vi "DHE_Settings.vi"(0 "refnum":i32, 1 "DHE_DBSRef":T1, 2 "raw args":string, 5 "Command":string, 7 "physical unit":string, 11 "error in (no error)":errorcluster, 12 "switches":string[](array[string]), 13 "switches args":string[](array[string])) -> (3 "message":string, 4 "refnum out":i32, 8 "Read Value":i32, 15 "error out":errorcluster)   [LabVIEW 2016]
uses:
  DBSHAND/private/vis/DatabaseHand_RefNum.ctl
  DBSHAND/private/vis/DatabaseHand_Element_Set(string).vi
  DBSHAND/private/vis/DatabaseHand_Element_Set(U32).vi
  DBSHAND/private/vis/DatabaseHand_Element_Set(bool).vi
  DBSHAND/private/vis/DatabaseHand_Element_Get(U16).vi
  DBSHAND/private/vis/DatabaseHand_Element_Set(U16).vi
  DBSHAND/private/vis/DatabaseHand_Element_Get(bool).vi
  DBSHAND/private/vis/DatabaseHand_Element_Set(double).vi
  DBSHAND/private/vis/DatabaseHand_Element_Set(I32).vi
  DBSHAND/private/vis/DatabaseHand_Element_Get(string).vi
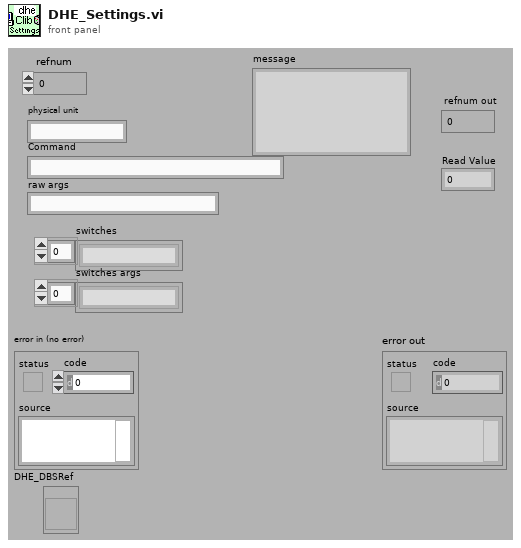
[diagram p1: front panel]
types:
  T1 = typedef "DatabaseHand_RefNum.ctl" = refnum<vi>
  T2 = enum16{"get", "send", "delete", "add", "clean", "send_all", "send_on", "send_off"}
  T3 = enum16{"add", "delete", "find", "clear all", "getall", "all"}
  T4 = enum16{"add", "delete", "find", "clear all", "getall"}
  T5 = typedef "CMN_ContStatus.ctl" = cluster{"Response":string, "power":bool, "shutter":bool, "artifdata":bool, "idlemode":bool, "reset":bool, "gain":u8, "speed":u8, "resetPCI":bool, "autoshutter":bool, "TempSetPoint":i32, "multipleextensions":bool, "displayImage":bool, "coadding":bool, "images being coadded":i32, "Operation Mode":enum16{"normal", "coadd", "fawler"}, "frames to write":cluster{"subs":bool, "reset":bool, "exposed":bool}, "fawler samples":i32, "write auto":bool, "datatype":string, "frames to display":cluster{"subs":bool, "reset":bool, "exposed":bool}, "sur":i32, "autoclear":bool}
  T6 = typedef "DHE_Img.ctl" = cluster{"title":string, "comment":string, "rootname":string, "imnumber":i32, "mext":bool, "imdir":string, "basename":string, "imprefix":string, "imsufix":string, "froot":string}
  T7 = typedef "DHE_Obs.ctl" = cluster{"observer":string, "obstype":string, "exptime":dbl, "coadds":i32, "fowler":i32, "nimages":i32, "display":bool, "autowrite":bool, "frames to write":cluster{"subs":bool, "reset":bool, "exposed":bool}, "frames to display":cluster{"subs":bool, "reset":bool, "exposed":bool}, "sur":i32}
  T8 = typedef "CMN_TimingInfo.ctl" = cluster{"PixelTime":sgl, "SkipPixel":sgl, "SkipRow":sgl, "ShiftRow":sgl, "ShiftedPix":u16, "known_overhead":sgl, "DET_READ_TIME":sgl}
  T9 = typedef "GEOM_CorrectedFPA.ctl" = cluster{"readmode":string, "amplifiers":cluster{"number":i32, "xstart":i32, "ystart":i32}[], "totxsize":i32, "totysize":i32, "maxxdim":i32, "maxydim":i32, "numxamps":i32, "numyamps":i32, "totxdata":i32, "totydata":i32, "xdataamp":i32, "ydataamp":i32, "totpixels":i32}
  T10 = typedef "GEOM_Amplifier.ctl" = cluster{"number":i32, "type":T11, "rotated":i16, "fliped":u16, "FPAcoord":cluster{"xstart":i32, "ystart":i32}, "Physical_size":cluster{"columns":i32, "rows":i32}, "predata":cluster{"columns":i32, "rows":i32}, "postdata":cluster{"columns":i32, "rows":i32}, "Req ROIs":T12, "Corr ROI":T12, "Detnumber":i32, "ampID":string, "discard":i32}
  T11 = typedef "GEOM_AmpType.ctl" = u16
  T12 = typedef "GEOM_ROI.ctl" = T13[]
  T13 = typedef "GEOM_Coords.ctl" = cluster{"xstart":u32, "ystart":u32, "xsize":u32, "ysize":u32}
  T14 = typedef "GEOM_AmpModifiers.ctl" = cluster{"Binning":T15, "sections":T16[]}
  T15 = typedef "GEOM_Binning.ctl" = cluster{"x":u32, "y":u32}
  T16 = typedef "GEOM_Moifier.ctl" = cluster{"name":string, "header section":string, "comment":string, "value":i32, "binning?":bool, "Where":enum16{"predata", "postdata"}, "add In":enum16{"columns", "rows", "none"}}
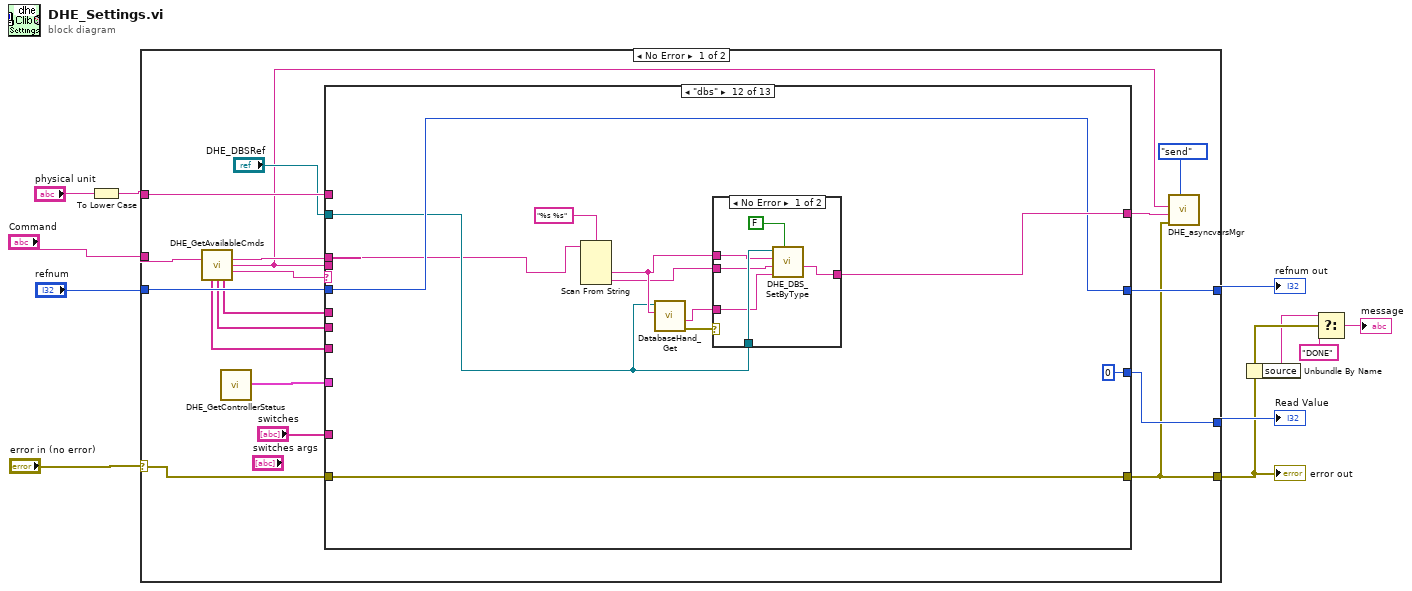
[diagram p0: block diagram]
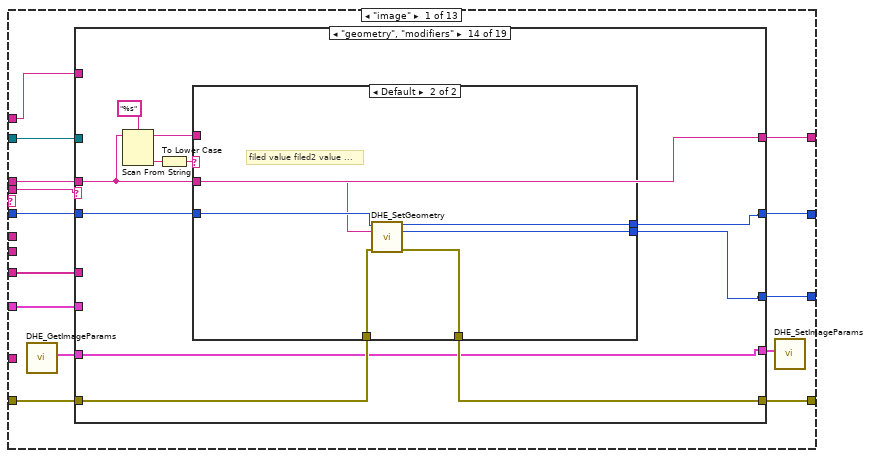
[diagram p2: hidden frame]
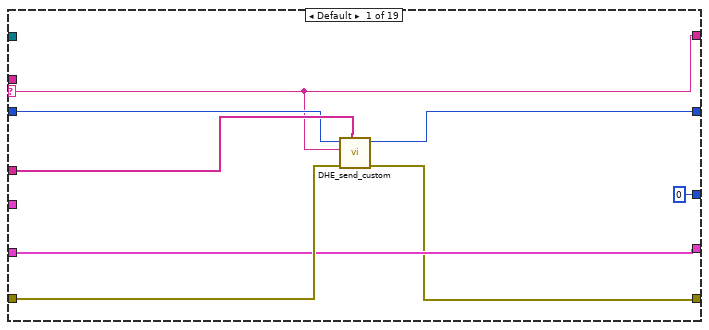
[diagram p3: hidden frame]
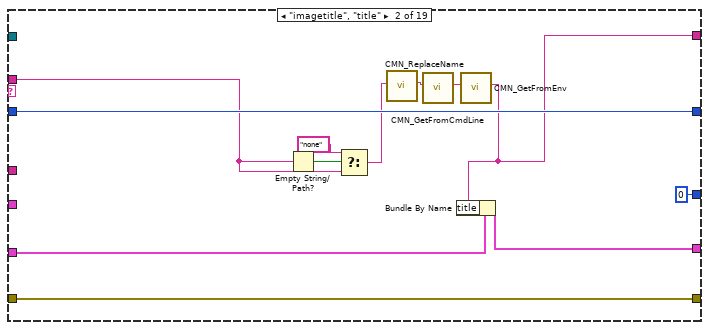
[diagram p4: hidden frame]
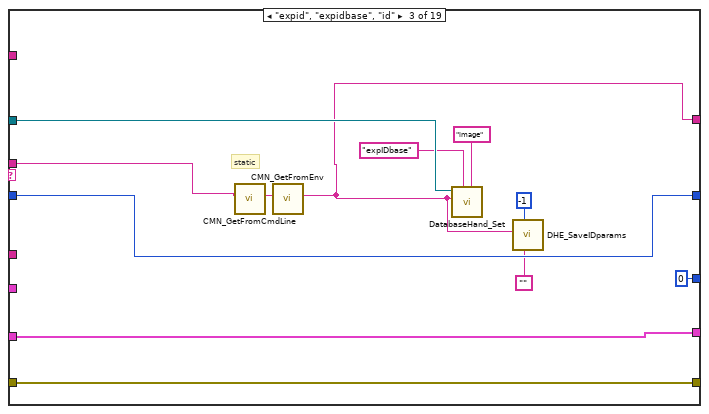
[diagram p5: hidden frame]
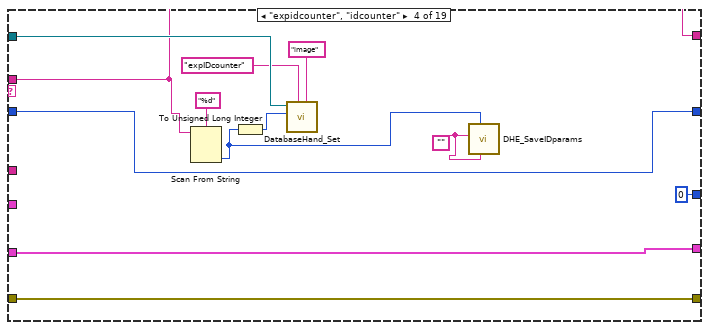
[diagram p6: hidden frame]
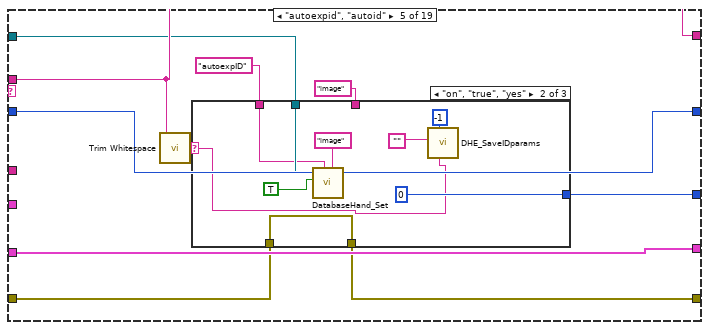
[diagram p7: hidden frame]
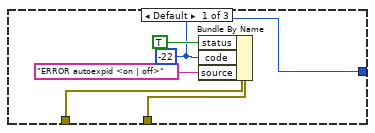
[diagram p8: hidden frame]
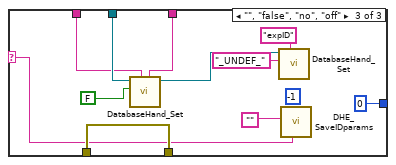
[diagram p9: hidden frame]
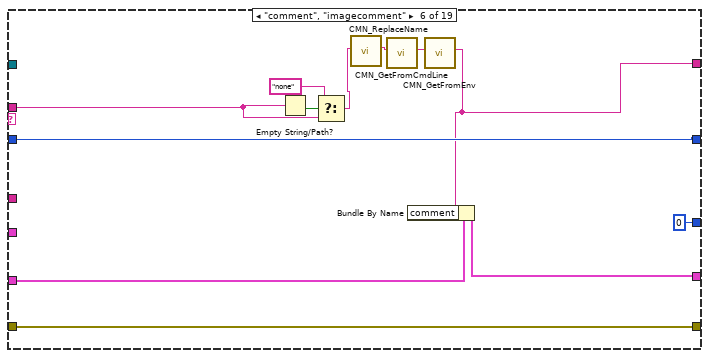
[diagram p10: hidden frame]
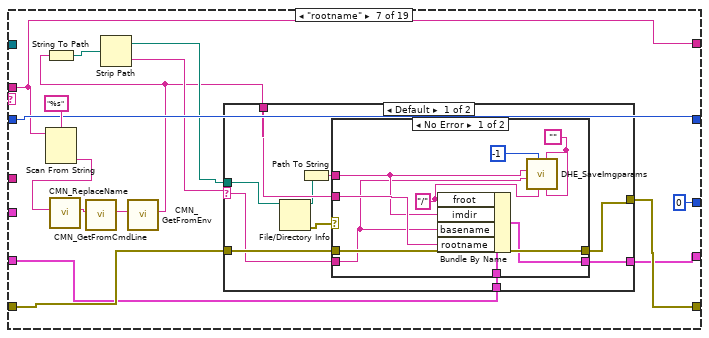
[diagram p11: hidden frame]
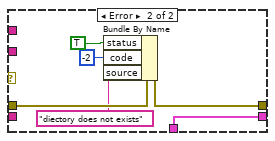
[diagram p12: hidden frame]
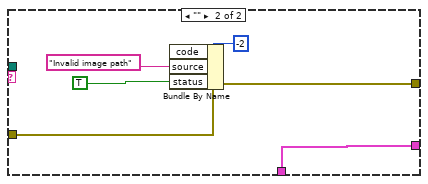
[diagram p13: hidden frame]
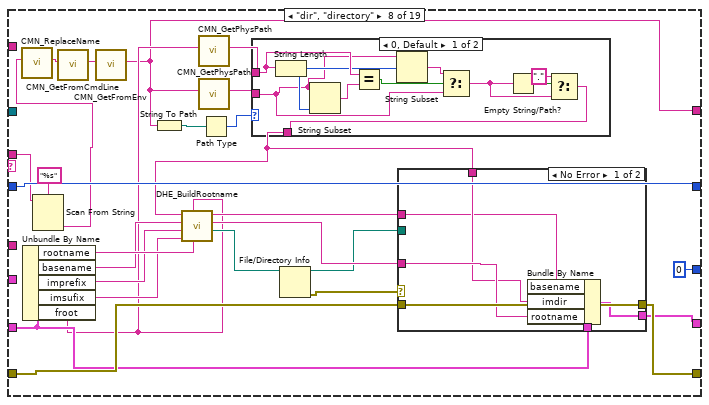
[diagram p14: hidden frame]
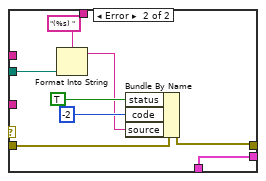
[diagram p16: hidden frame]
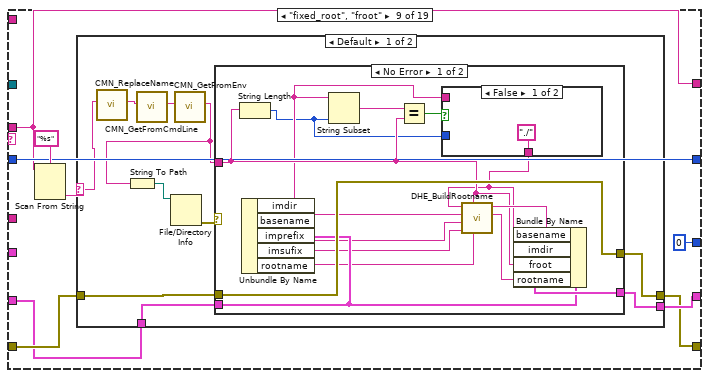
[diagram p17: hidden frame]
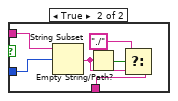
[diagram p18: hidden frame]
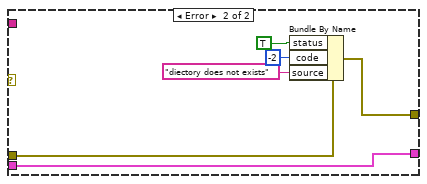
[diagram p19: hidden frame]
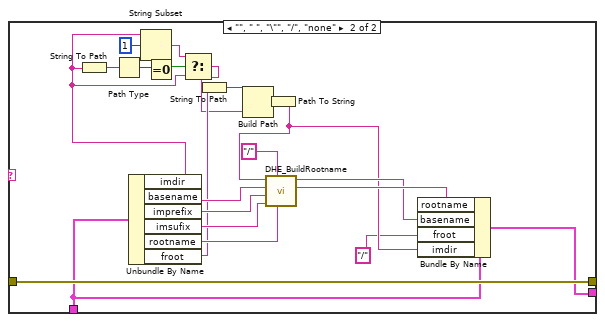
[diagram p20: hidden frame]
diagram:
  n1 = To Lower Case(string="physical unit") -> (all lower case string=w6:string)
  n2 = case shown="No Error" "error in (no error)" {
    selector: "error in (no error)" -> [w24 w2013]
    tunnel: [w14 w2013] -> w4
    tunnel: "refnum" -> [w29 w2015]
    tunnel: [w28 w2015] -> w10
    tunnel: "Command" -> [w23 _]
    tunnel: [w27 w2014] -> w11
    tunnel: w6 -> [w25 _]
    frame No Error {
      n3 = call "DHE_GetAvailableCmds.vi"("input command"=w23) -> ("remaining"=w18:string, "field"=w13:string, "parent"=w19:string, "SDSU_image_cmds out"=w20:string[], "SDSU_dhe_cmds out"=w21:string[], "SDSU_obs_cmds out"=w22:string[])  [unwired: 9 out]
      n4 = call "DHE_GetControllerStatus.vi"() -> ("ControllerStatus"=w26:T5)  [unwired: 11 out]
      n5 = case shown="\"dbs\"" w19 {
        selector: w19 -> [_ _ _ _ _ _ _ _ _ _ _ _ w1992]
        tunnel: w24 -> [w40 w617 w1252 w1806 w1831 w1833 w1843 w1854 w1889 w1940 w1942 w1974 w1999]
        tunnel: [w39 w609 w1248 w1805 w1831 w1833 w1843 w1853 w1885 w1940 w1941 w1974 w1989] -> w14
        tunnel: w29 -> [w38 w619 w1251 w1803 w1830 w1834 w1844 w1851 w1891 w1939 w1950 w1975 w1996]
        tunnel: [w37 w618 w1250 w1803 w1830 w1834 w1844 w1851 w1887 w1939 w1950 w1975 w1995] -> w28
        tunnel: [w43 w620 w1249 w1804 u32 0 ("code") u32 0 ("code") u32 0 ("code") w1852 w1886 u32 0 ("code") u32 0 ("code") u32 0 ("code") w1998] -> w27
        tunnel: w18 -> [w42 w621 w1247 w1808 w1827 w1836 w1846 w1850 w1883 w1935 w1948 w1971 w1994]
        tunnel: w26 -> [w35 w614 w1244 w1800 _ _ _ _ _ _ _ _ _]
        tunnel: w25 -> [w30 w615 _ _ _ _ _ _ _ _ _ _ _]
        tunnel: w22 -> [_ w616 _ _ _ _ _ _ _ _ _ _ _]
        tunnel: w21 -> [_ _ w1245 _ _ _ _ _ _ _ _ _ _]
        tunnel: w20 -> [w36 _ _ _ _ _ _ _ _ _ _ _ _]
        tunnel: w13 -> [w41 w610 w1246 _ _ _ _ _ _ _ _ _ _]
        tunnel: "DHE_DBSRef" -> [w31 w611 w1243 _ _ _ _ w1855 w1890 w1932 _ w1972 _]
        tunnel: "switches" -> [_ w607 _ _ _ _ _ _ w1884 _ _ _ _]
        tunnel: [w32 w608 w1242 w1799 "" w1832 w1842 w1850 w1883 w1935 w1943 w1976 w1992] -> w12
        frame "image" {
          n6 = call "DHE_GetImageParams.vi"() -> ("DHE_IMAGE"=w34:T6)  [unwired: 11 out]
          n7 = case shown="\"geometry\", \"modifiers\"" w41 {
            selector: w41 -> [w44 _ _ _ _ _ _ _ _ _ _ _ _ _ _ _ _ _ _]
            tunnel: [u32 0 ("code") u32 0 ("code") u32 0 ("code") u32 0 ("code") w89 u32 0 ("code") u32 0 ("code") u32 0 ("code") u32 0 ("code") u32 0 ("code") u32 0 ("code") u32 0 ("code") u32 0 ("code") w412 w437 w452 w493 w530 u32 0 ("code")] -> w43
            tunnel: w42 -> [_ w56 w64 w80 w95 w125 w139 w185 w233 w306 w348 w379 w400 w410 _ w449 w491 w534 w594]
            tunnel: w40 -> [w51 w62 w74 w86 w92 w134 w146 w205 w239 w320 w351 w382 w405 w416 w439 w444 w486 w532 w592]
            tunnel: [w45 w62 w74 w86 w91 w134 w145 w204 w234 w319 w350 w381 w405 w415 w438 w443 w485 w531 w592] -> w39
            tunnel: w38 -> [w47 w61 w72 w84 w97 w132 w147 w206 w237 w321 w352 w383 w403 w414 w436 w451 w492 w528 w589]
            tunnel: [w46 w61 w72 w84 w97 w132 w147 w206 w237 w321 w352 w383 w403 w413 w436 w451 w492 w529 w589] -> w37
            tunnel: w36 -> [w49 _ _ _ _ _ _ _ _ _ _ _ _ _ _ _ _ _ _]
            tunnel: w35 -> [_ _ _ _ _ _ _ _ _ _ _ _ _ _ _ w453 _ _ _]
            tunnel: w34 -> [w48 w60 w69 w81 w96 w131 w143 w201 w238 w316 w346 w377 w402 w411 w435 w448 w488 w527 w591]
            tunnel: [w48 w59 w69 w81 w96 w130 w142 w202 w235 w317 w347 w378 w401 w411 w435 w450 w488 w527 w591] -> w33
            tunnel: [w44 w52 w67 w80 w95 w123 w139 w181 w233 w302 w334 w365 w400 w410 "" ("remaining") w442 w490 w533 w588] -> w32
            tunnel: w31 -> [_ _ w71 w83 w94 _ _ _ _ _ _ _ _ _ _ w445 w489 w536 w585]
            tunnel: w30 -> [_ _ _ _ _ _ _ _ _ _ _ _ _ _ _ _ _ w535 w593]
            frame Default {
              n8 = call "DHE_send_custom.vi"("valid params"=w49, "error in (no error)"=w51, "args"=w44, "fd"=w47) -> ("error IO"=w45:errorcluster, "fd out"=w46:i32)  [unwired: 6 out]
            }
            frame "imagetitle", "title" {
              n9 = Empty String/Path?(string/path=w56) -> (empty?=w58:bool)
              n10 = Select(t="none", s=w58, f=w56) -> (s? t:f=w53:string)
              n11 = call "CMN_ReplaceName.vi"("name in"=w53) -> ("name out"=w54:string)  [unwired: 1 in, 9 out]
              n12 = call "CMN_GetFromCmdLine.vi"("str in"=w54) -> ("str out"=w55:string)  [unwired: 10 out]
              n13 = call "CMN_GetFromEnv.vi"("str in"=w55) -> ("str out"=w52:string)  [unwired: 10 out]
              n14 = Bundle By Name(cluster=w60, "title"=w52) -> (w59:T6)
            }
            frame "expid", "expidbase", "id" {
              # "static"
              n15 = call "CMN_GetFromCmdLine.vi"("str in"=w64) -> ("str out"=w68:string)  [unwired: 10 out]
              n16 = call "CMN_GetFromEnv.vi"("str in"=w68) -> ("str out"=w67:string)  [unwired: 10 out]
              n17 = call-poly "DatabaseHand_Set.vi"("group"="image", "name"="expIDbase" ("value"), "value"=w67, "Database RefNum in"=w71) -> ()  [unwired: 4 in, 4 out]
              n18 = call "DHE_SaveIDparams.vi"("autoid"="", "expidcounter"=-1, "expidbase"=w67) -> ()  [unwired: 9 out]
            }
            frame "expidcounter", "idcounter" {
              w78 = ""
              n19 = Scan From String(format string="%d", input string=w80) -> (output 1=w76:i32)  [unwired: 2 in, 4 out]
              n20 = To Unsigned Long Integer(number=w76) -> (unsigned 32bit integer=w77:u32)
              n21 = call-poly "DatabaseHand_Set.vi"("group"="image", "name"="expIDcounter" ("value"), "value"=w77, "Database RefNum in"=w83) -> ()  [unwired: 4 in, 4 out]
              n22 = call "DHE_SaveIDparams.vi"("autoid"=w78, "expidcounter"=w76, "expidbase"=w78) -> ()  [unwired: 9 out]
            }
            frame "autoexpid", "autoid" {
              n23 = call <vilib>:"Trim Whitespace.vi"("string"=w95) -> ("trimmed string"=w88:string)  [unwired: 1 in]
              n24 = case shown="\"on\", \"true\", \"yes\"" w88 {
                selector: w88 -> [_ w104 w112]
                tunnel: w94 -> [_ w110 w122]
                tunnel: "autoexpID" ("value") -> [_ w108 w120]
                tunnel: w92 -> [w102 w107 w119]
                tunnel: [w101 w107 w119] -> w91
                tunnel: "image" ("group") -> [_ _ w118]
                tunnel: [w98 0 ("code") 0 ("code")] -> w89
                frame Default {
                  w98 = -22 ("code")
                  n25 = Bundle By Name(cluster=w102, "status"=TRUE, "code"=w98, "source"="ERROR autoexpid <on | off>") -> (w101:errorcluster)
                }
                frame "on", "true", "yes" {
                  n26 = call-poly "DatabaseHand_Set.vi"("group"="image", "name"=w108, "value"=TRUE, "Database RefNum in"=w110) -> ()  [unwired: 4 in, 4 out]
                  n27 = call "DHE_SaveIDparams.vi"("autoid"=w104, "expidcounter"=-1, "expidbase"="") -> ()  [unwired: 9 out]
                }
                frame "", "false", "no", "off" {
                  (unwired) -1 ("expidcounter")
                  n28 = call-poly "DatabaseHand_Set.vi"("group"=w118, "name"=w120, "value"=FALSE, "Database RefNum in"=w122) -> ("Database RefNum out"=w116:T1)  [unwired: 4 in, 3 out]
                  n29 = call-poly "DatabaseHand_Set.vi"("name"="expID", "value"="_UNDEF_", "Database RefNum in"=w116) -> ()  [unwired: 5 in, 4 out]
                  n30 = call "DHE_SaveIDparams.vi"("autoid"=w112, "expidbase"="") -> ()  [unwired: 1 in, 9 out]
                }
              }
            }
            frame "comment", "imagecomment" {
              n31 = Empty String/Path?(string/path=w125) -> (empty?=w129:bool)
              n32 = Select(t="none", s=w129, f=w125) -> (s? t:f=w124:string)
              n33 = call "CMN_ReplaceName.vi"("name in"=w124) -> ("name out"=w126:string)  [unwired: 1 in, 9 out]
              n34 = call "CMN_GetFromCmdLine.vi"("str in"=w126) -> ("str out"=w127:string)  [unwired: 10 out]
              n35 = call "CMN_GetFromEnv.vi"("str in"=w127) -> ("str out"=w123:string)  [unwired: 10 out]
              n36 = Bundle By Name(cluster=w131, "comment"=w123) -> (w130:T6)
            }
            frame "rootname" {
              n37 = Scan From String(format string="%s", input string=w139) -> (output 1=w136:string)  [unwired: 2 in, 4 out]
              n38 = call "CMN_ReplaceName.vi"("name in"=w136) -> ("name out"=w137:string)  [unwired: 1 in, 9 out]
              n39 = call "CMN_GetFromCmdLine.vi"("str in"=w137) -> ("str out"=w138:string)  [unwired: 10 out]
              n40 = call "CMN_GetFromEnv.vi"("str in"=w138) -> ("str out"=w135:string)  [unwired: 10 out]
              n41 = String To Path(string=w135) -> (path=w149:path)
              n42 = Strip Path(path=w149) -> (stripped path=w141:path, name=w140:string)
              n43 = case shown="Default" w140 {
                selector: w140 -> [w150 _]
                tunnel: w135 -> [w159 _]
                tunnel: w146 -> [w158 w180]
                tunnel: [w157 w179] -> w145
                tunnel: w141 -> [w156 _]
                tunnel: w143 -> [w154 w176]
                tunnel: [w153 w176] -> w142
                frame Default {
                  n44 = File/Directory Info(path=w156) -> (path out=w152:path, error out=w155:errorcluster)  [unwired: 1 in, 5 out]
                  n45 = Path To String(path=w152) -> (string=w151:string)
                  n46 = case shown="No Error" w155 {
                    tunnel: w159 -> [w165 _]
                    tunnel: w158 -> [w168 w174]
                    tunnel: [w168 w173] -> w157
                    tunnel: w154 -> [w167 w169]
                    tunnel: [w166 w169] -> w153
                    tunnel: w151 -> [w162 _]
                    tunnel: w150 -> [w161 _]
                    frame No Error {
                      w163 = ""
                      w160 = "/" ("froot")
                      n47 = Bundle By Name(cluster=w167, "froot"=w160, "imdir"=w162, "basename"=w161, "rootname"=w165) -> (w166:T6)
                      n48 = call "DHE_SaveImgparams.vi"("prefix"=w163, "sufix"=w163, "froot"=w160, "number"=-1, "basename"=w161, "dir"=w162) -> ()  [unwired: 6 out]
                    }
                    frame Error {
                      n49 = Bundle By Name(cluster=w174, "status"=TRUE, "code"=-2, "source"="diectory does not exists") -> (w173:errorcluster)
                    }
                  }
                }
                frame "" {
                  n50 = Bundle By Name(cluster=w180, "code"=-2, "source"="Invalid image path", "status"=TRUE) -> (w179:errorcluster)
                }
              }
            }
            frame "dir", "directory" {
              n51 = Unbundle By Name(w201) -> ("rootname"=w199:string, "basename"=w198:string, "imprefix"=w197:string, "imsufix"=w196:string, "froot"=w186:string)
              n52 = Scan From String(format string="%s", input string=w185) -> (output 1=w182:string)  [unwired: 2 in, 4 out]
              n53 = call "CMN_ReplaceName.vi"("name in"=w182) -> ("name out"=w183:string)  [unwired: 1 in, 9 out]
              n54 = call "CMN_GetFromCmdLine.vi"("str in"=w183) -> ("str out"=w184:string)  [unwired: 10 out]
              n55 = call "CMN_GetFromEnv.vi"("str in"=w184) -> ("str out"=w181:string)  [unwired: 10 out]
              n56 = String To Path(string=w181) -> (path=w190:path)
              n57 = call "CMN_GetPhysPath.vi"("path"=w186) -> ("physical path"=w192:string)  [unwired: 10 out]
              n58 = call "CMN_GetPhysPath.vi"("path"=w181) -> ("physical path"=w191:string)  [unwired: 10 out]
              n59 = Path Type(1:w190) -> (0:w189:i16)
              n60 = case shown="0, Default" w189 {
                tunnel: w191 -> [w212 w218]
                tunnel: [w209 w218] -> w187
                tunnel: w192 -> [w217 _]
                frame 0, Default {
                  n61 = String Length(string=w217) -> (length=w214:i32)
                  n62 = String Subset(string=w212, length (rest)=w214) -> (substring=w216:string)  [unwired: 1 out]
                  n63 = Equal?(x=w217, y=w216) -> (x = y?=w215:bool)
                  n64 = String Subset(string=w212, offset (0)=w214) -> (substring=w213:string)  [unwired: 1 out]
                  n65 = Select(t=w213, s=w215, f=w212) -> (s? t:f=w210:string)
                  n66 = Empty String/Path?(string/path=w210) -> (empty?=w211:bool)
                  n67 = Select(t=".", s=w211, f=w210) -> (s? t:f=w209:string)
                }
                frame 1 {
                }
              }
              n68 = call "DHE_BuildRootname.vi"("orig rootname"=w199, "froot"=w186, "sufix"=w196, "prefix"=w197, "basename"=w198, "imdir"=w187) -> ("rootpath"=w195:path, "rootname"=w194:string, "basename out"=w193:string)  [unwired: 2 out]
              n69 = File/Directory Info(path=w195) -> (path out=w188:path, error out=w200:errorcluster)  [unwired: 1 in, 5 out]
              n70 = case shown="No Error" w200 {
                tunnel: w194 -> [w221 _]
                tunnel: w205 -> [w224 w227]
                tunnel: [w224 w226] -> w204
                tunnel: w201 -> [w223 w232]
                tunnel: [w222 w232] -> w202
                tunnel: w187 -> [w220 _]
                tunnel: w193 -> [w219 _]
                tunnel: w188 -> [_ w225]
                frame No Error {
                  n71 = Bundle By Name(cluster=w223, "basename"=w219, "imdir"=w220, "rootname"=w221) -> (w222:T6)
                }
                frame Error {
                  n72 = Format Into String(format string="(%s) " ("source"), w225) -> (resulting string=w228:string)  [unwired: 2 in, 1 out]
                  n73 = Bundle By Name(cluster=w227, "status"=TRUE, "code"=-2, "source"=w228) -> (w226:errorcluster)
                }
              }
            }
            frame "fixed_root", "froot" {
              n74 = Scan From String(format string="%s", input string=w233) -> (output 1=w240:string)  [unwired: 2 in, 4 out]
              n75 = case shown="Default" w240 {
                selector: w240 -> [w243 _]
                tunnel: w239 -> [w247 w301]
                tunnel: [w246 w301] -> w234
                tunnel: w238 -> [w251 w296]
                tunnel: [w250 w293] -> w235
                frame Default {
                  n76 = call "CMN_ReplaceName.vi"("name in"=w243) -> ("name out"=w244:string)  [unwired: 1 in, 9 out]
                  n77 = call "CMN_GetFromCmdLine.vi"("str in"=w244) -> ("str out"=w245:string)  [unwired: 10 out]
                  n78 = call "CMN_GetFromEnv.vi"("str in"=w245) -> ("str out"=w242:string)  [unwired: 10 out]
                  n79 = String To Path(string=w242) -> (path=w249:path)
                  n80 = File/Directory Info(path=w249) -> (error out=w248:errorcluster)  [unwired: 1 in, 6 out]
                  n81 = case shown="No Error" w248 {
                    tunnel: w251 -> [w264 w274]
                    tunnel: [w266 w274] -> w250
                    tunnel: w247 -> [w265 w276]
                    tunnel: [w265 w275] -> w246
                    tunnel: w242 -> [w256 _]
                    frame No Error {
                      n82 = String Length(string=w256) -> (length=w252:i32)
                      n83 = Unbundle By Name(w264) -> ("imdir"=w253:string, "basename"=w260:string, "imprefix"=w261:string, "imsufix"=w262:string, "rootname"=w263:string)
                      n84 = String Subset(string=w253, length (rest)=w252) -> (substring=w257:string)  [unwired: 1 out]
                      n85 = Equal?(x=w257, y=w256) -> (x = y?=w255:bool)
                      n86 = case shown="False" w255 {
                        tunnel: ["./" w269] -> w254
                        tunnel: w253 -> [_ w273]
                        tunnel: w252 -> [_ w272]
                        frame False {
                        }
                        frame True {
                          n87 = String Subset(string=w273, offset (0)=w272) -> (substring=w270:string)  [unwired: 1 out]
                          n88 = Empty String/Path?(string/path=w270) -> (empty?=w271:bool)
                          n89 = Select(t="./", s=w271, f=w270) -> (s? t:f=w269:string)
                        }
                      }
                      n90 = call "DHE_BuildRootname.vi"("orig rootname"=w263, "froot"=w256, "sufix"=w262, "prefix"=w261, "basename"=w260, "imdir"=w254) -> ("rootname"=w259:string, "basename out"=w258:string)  [unwired: 3 out]
                      n91 = Bundle By Name(cluster=w264, "basename"=w258, "imdir"=w254, "froot"=w256, "rootname"=w259) -> (w266:T6)
                    }
                    frame Error {
                      n92 = Bundle By Name(cluster=w276, "status"=TRUE, "code"=-2, "source"="diectory does not exists") -> (w275:errorcluster)
                    }
                  }
                }
                frame "", " ", "\"", "/", "none" {
                  n93 = Unbundle By Name(w296) -> ("imdir"=w282:string, "basename"=w300:string, "imprefix"=w299:string, "imsufix"=w298:string, "rootname"=w297:string, "froot"=w292:string)
                  n94 = String To Path(string=w282) -> (path=w286:path)
                  n95 = Path Type(1:w286) -> (0:w285:i16)
                  n96 = String Subset(string=w282, offset (0)=1) -> (substring=w280:string)  [unwired: 1 out]
                  n97 = Equal To 0?(x=w285) -> (x = 0?=w284:bool)
                  n98 = Select(t=w280, s=w284, f=w282) -> (s? t:f=w283:string)
                  n99 = String To Path(string=w292) -> (path=w291:path)
                  n100 = Build Path(base path=w291, name or relative path=w283) -> (appended path=w290:path)
                  n101 = Path To String(path=w290) -> (string=w289:string)
                  n102 = call "DHE_BuildRootname.vi"("orig rootname"=w297, "froot"="/", "sufix"=w298, "prefix"=w299, "basename"=w300, "imdir"=w289) -> ("rootname"=w295:string, "basename out"=w294:string)  [unwired: 3 out]
                  n103 = Bundle By Name(cluster=w296, "rootname"=w295, "basename"=w294, "froot"="/", "imdir"=w289) -> (w293:T6)
                }
              }
            }
            frame "basename" {
              n104 = Unbundle By Name(w316) -> ("rootname"=w314:string, "imdir"=w313:string, "imprefix"=w312:string, "imsufix"=w311:string, "froot"=w308:string)
              n105 = Scan From String(format string="%s", input string=w306) -> (output 1=w303:string)  [unwired: 2 in, 4 out]
              n106 = call "CMN_ReplaceName.vi"("name in"=w303) -> ("name out"=w304:string)  [unwired: 1 in, 9 out]
              n107 = call "CMN_GetFromCmdLine.vi"("str in"=w304) -> ("str out"=w305:string)  [unwired: 10 out]
              n108 = call "CMN_GetFromEnv.vi"("str in"=w305) -> ("str out"=w302:string)  [unwired: 10 out]
              n109 = call "DHE_BuildRootname.vi"("orig rootname"=w314, "froot"=w308, "sufix"=w311, "prefix"=w312, "basename"=w302, "imdir"=w313) -> ("rootpath"=w310:path, "rootname"=w309:string, "basename out"=w307:string)  [unwired: 2 out]
              n110 = File/Directory Info(path=w310) -> (error out=w315:errorcluster)  [unwired: 1 in, 6 out]
              n111 = case shown="No Error" w315 {
                tunnel: w320 -> [w327 w333]
                tunnel: [w327 w332] -> w319
                tunnel: w316 -> [w326 w328]
                tunnel: [w325 w328] -> w317
                tunnel: w309 -> [w324 _]
                tunnel: w307 -> [w323 _]
                frame No Error {
                  n112 = Bundle By Name(cluster=w326, "basename"=w323, "rootname"=w324) -> (w325:T6)
                }
                frame Error {
                  n113 = Bundle By Name(cluster=w333, "status"=TRUE, "code"=-2, "source"="diectory does not exists") -> (w332:errorcluster)
                }
              }
            }
            frame "imprefix", "prefix" {
              n114 = Unbundle By Name(w346) -> ("rootname"=w344:string, "imdir"=w343:string, "basename"=w339:string, "imsufix"=w342:string, "froot"=w338:string)
              n115 = Scan From String(format string="%s", input string=w348) -> (output 1=w335:string)  [unwired: 2 in, 4 out]
              n116 = call "CMN_ReplaceName.vi"("name in"=w335) -> ("name out"=w336:string)  [unwired: 1 in, 9 out]
              n117 = call "CMN_GetFromCmdLine.vi"("str in"=w336) -> ("str out"=w337:string)  [unwired: 10 out]
              n118 = call "CMN_GetFromEnv.vi"("str in"=w337) -> ("str out"=w334:string)  [unwired: 10 out]
              n119 = call "DHE_BuildRootname.vi"("orig rootname"=w344, "froot"=w338, "sufix"=w342, "prefix"=w335, "basename"=w339, "imdir"=w343) -> ("rootpath"=w341:path, "rootname"=w340:string)  [unwired: 3 out]
              n120 = File/Directory Info(path=w341) -> (error out=w345:errorcluster)  [unwired: 1 in, 6 out]
              n121 = case shown="No Error" w345 {
                tunnel: w351 -> [w358 w364]
                tunnel: [w358 w363] -> w350
                tunnel: w346 -> [w357 w359]
                tunnel: [w356 w359] -> w347
                tunnel: w340 -> [w355 _]
                tunnel: w334 -> [w354 _]
                frame No Error {
                  n122 = Bundle By Name(cluster=w357, "imprefix"=w354, "rootname"=w355) -> (w356:T6)
                }
                frame Error {
                  n123 = Bundle By Name(cluster=w364, "status"=TRUE, "code"=-2, "source"="diectory does not exists") -> (w363:errorcluster)
                }
              }
            }
            frame "imsufix", "sufix" {
              n124 = Unbundle By Name(w377) -> ("rootname"=w375:string, "imdir"=w374:string, "basename"=w371:string, "imprefix"=w370:string, "froot"=w369:string)
              n125 = Scan From String(format string="%s", input string=w379) -> (output 1=w366:string)  [unwired: 2 in, 4 out]
              n126 = call "CMN_ReplaceName.vi"("name in"=w366) -> ("name out"=w367:string)  [unwired: 1 in, 9 out]
              n127 = call "CMN_GetFromCmdLine.vi"("str in"=w367) -> ("str out"=w368:string)  [unwired: 10 out]
              n128 = call "DHE_BuildRootname.vi"("orig rootname"=w375, "froot"=w369, "sufix"=w366, "prefix"=w370, "basename"=w371, "imdir"=w374) -> ("rootpath"=w373:path, "rootname"=w372:string)  [unwired: 3 out]
              n129 = call "CMN_GetFromEnv.vi"("str in"=w368) -> ("str out"=w365:string)  [unwired: 10 out]
              n130 = File/Directory Info(path=w373) -> (error out=w376:errorcluster)  [unwired: 1 in, 6 out]
              n131 = case shown="No Error" w376 {
                tunnel: w382 -> [w389 w395]
                tunnel: [w389 w394] -> w381
                tunnel: w377 -> [w388 w390]
                tunnel: [w387 w390] -> w378
                tunnel: w372 -> [w386 _]
                tunnel: w365 -> [w385 _]
                frame No Error {
                  n132 = Bundle By Name(cluster=w388, "imsufix"=w385, "rootname"=w386) -> (w387:T6)
                }
                frame Error {
                  n133 = Bundle By Name(cluster=w395, "status"=TRUE, "code"=-2, "source"="diectory does not exists") -> (w394:errorcluster)
                }
              }
            }
            frame "imagenumber", "imnumber", "number" {
              w396 = ""
              n134 = Decimal String To Number(string=w400) -> (number=w398:i32)  [unwired: 3 out]
              n135 = Max & Min(x=w398, y=0) -> (max(x,y)=w397:i32)  [unwired: 1 out]
              n136 = call "DHE_SaveImgparams.vi"("prefix"=w396, "sufix"=w396, "froot"=w396, "number"=w397, "basename"=w396, "dir"=w396) -> ()  [unwired: 6 out]
              n137 = Bundle By Name(cluster=w402, "imnumber"=w397) -> (w401:T6)
            }
            frame "geometry", "modifiers" {
              n138 = Scan From String(format string="%s", input string=w410) -> (remaining string=w406:string, output 1=w408:string)  [unwired: 2 in, 3 out]
              n139 = To Lower Case(string=w408) -> (all lower case string=w407:string)
              n140 = case shown="Default" w407 {
                selector: w407 -> [w417 _]
                tunnel: w416 -> [w427 w433]
                tunnel: [w427 w432] -> w415
                tunnel: w414 -> [w426 w431]
                tunnel: [w426 w430] -> w413
                tunnel: [0 ("return value") w429] -> w412
                tunnel: w410 -> [_ w428]
                tunnel: w406 -> [w420 _]
                frame "order", "xorder", "yorder" {
                  n141 = Concatenate Strings("SET " ("command"), w417, w420) -> (w419:string)
                  n142 = call "CMN_toUnsc.vi"("responseQ"="dhe2unsc", "ms timeout (-1)"=5000, "command"=w419) -> ("error out"=w423:errorcluster)  [unwired: 6 in, 2 out]
                  n143 = call "GEOM_CallGeometry.vi"("Command"="GET HEADER", "error in (no error)"=w423) -> ()  [unwired: 14 out]
                }
                frame Default {
                  # "filed value filed2 value ..."
                  n144 = call "DHE_SetGeometry.vi"("refnum"=w431, "modifiers"=w428, "error in (no error)"=w433) -> ("fd out"=w430:i32, "return value"=w429:i32, "error out"=w432:errorcluster)  [unwired: 10 out]
                }
              }
            }
            frame "progress" {
              w437 = -1 ("code")
              n145 = Bundle By Name(cluster=w439, "status"=TRUE, "code"=w437, "source"="ERR: read-only parameter") -> (w438:errorcluster)
            }
            frame "extensions", "mext", "multipleextensions" {
              n146 = call <vilib>:"Trim Whitespace.vi"("string"=w449) -> ("trimmed string"=w446:string)  [unwired: 1 in]
              n147 = To Lower Case(string=w446) -> (all lower case string=w442:string)
              n148 = case shown="\"on\", \"true\", \"yes\"" w442 {
                tunnel: [w455 TRUE w475] -> w447
                tunnel: w444 -> [w459 w468 w477]
                tunnel: [w460 w468 w477] -> w443
                tunnel: w448 -> [w461 _ _]
                tunnel: w445 -> [_ w467 w473]
                frame Default {
                  n149 = Unbundle By Name(w461) -> ("mext"=w455:bool)
                  n150 = Bundle By Name(cluster=w459, "status"=TRUE, "code"=-22, "source"="ERROR <yes | no>") -> (w460:errorcluster)
                }
                frame "on", "true", "yes" {
                  n151 = call-poly "DatabaseHand_Get.vi"("default value"=u16 0, "name"="totnamps", "Database RefNum in"=w467) -> ("value"=w462:u16, "Database RefNum out"=w466:T1)  [unwired: 2 in, 5 out]
                  n152 = call-poly "DatabaseHand_Set.vi"("name"="num_ext", "value"=w462, "Database RefNum in"=w466) -> ()  [unwired: 5 in, 4 out]
                }
                frame "false", "no", "off" {
                  w476 = "detext" ("value")
                  w475 = FALSE
                  n153 = call-poly "DatabaseHand_Get.vi"("default value"=w475, "name"=w476, "Database RefNum in"=w473) -> ("value"=w474:bool)  [unwired: 2 in, 6 out]
                  n154 = call-poly "DatabaseHand_Set.vi"("name"="num_ext", "value"=u16 0, "Database RefNum in"=w473) -> ("Database RefNum out"=w472:T1)  [unwired: 5 in, 3 out]
                  n155 = case shown="True" w474 {
                    tunnel: w475 -> [_ w483]
                    tunnel: w472 -> [_ w481]
                    tunnel: w476 -> [_ w480]
                    frame False {
                    }
                    frame True {
                      n156 = call-poly "DatabaseHand_Set.vi"("name"=w480, "value"=w483, "Database RefNum in"=w481) -> ("error out"=w478:errorcluster)  [unwired: 5 in, 3 out]
                      n157 = call "GEOM_CallGeometry.vi"("Command"="GET HEADER", "error in (no error)"=w478) -> ("error out"=w482:errorcluster)  [unwired: 13 out]
                      n158 = stacked-sequence {
                        tunnel: w482 -> [_]
                        frame #0 {
                          n159 = call "CMN_toUnsc.vi"("command"="INIT") -> ()  [unwired: 8 in, 3 out]
                        }
                      }
                    }
                  }
                }
              }
              n160 = Bundle By Name(cluster=w453, "multipleextensions"=w447) -> (w454:T5)
              n161 = call "DHE_SetControllerParams.vi"("ControllerStatus"=w454) -> ()  [unwired: 1 in, 10 out]
              n162 = Bundle By Name(cluster=w448, "mext"=w447) -> (w450:T6)
              n163 = Unbundle By Name(w443) -> ("code"=w452:i32)
            }
            frame "detext" {
              n164 = call <vilib>:"Trim Whitespace.vi"("string"=w491) -> ("trimmed string"=w490:string)  [unwired: 1 in]
              n165 = Unbundle By Name(w488) -> ("mext"=w487:bool)
              n166 = case shown="True" w487 {
                tunnel: w486 -> [w495 w502]
                tunnel: w490 -> [_ w501]
                tunnel: w489 -> [_ w500]
                tunnel: [w494 w499] -> w485
                frame False {
                  n167 = Bundle By Name(cluster=w495, "status"=TRUE, "code"=-22, "source"="ERROR multiple extensions must be unabled; ignored.") -> (w494:errorcluster)
                }
                frame True {
                  n168 = case shown="\"on\", \"true\", \"yes\"" w501 {
                    tunnel: w502 -> [w506 _ w525]
                    tunnel: [w507 w508 w525] -> w499
                    tunnel: w500 -> [_ w513 w522]
                    frame Default {
                      n169 = Bundle By Name(cluster=w506, "status"=TRUE, "code"=-22, "source"="ERROR <yes | no>") -> (w507:errorcluster)
                    }
                    frame "on", "true", "yes" {
                      n170 = call-poly "DatabaseHand_Set.vi"("name"="detext" ("value"), "value"=TRUE, "Database RefNum in"=w513) -> ("error out"=w510:errorcluster)  [unwired: 5 in, 3 out]
                      n171 = call "GEOM_CallGeometry.vi"("Command"="GET HEADER", "error in (no error)"=w510) -> ("error out"=w509:errorcluster)  [unwired: 13 out]
                      n172 = stacked-sequence {
                        tunnel: w509 -> [_]
                        tunnel: [w515] -> w508
                        frame #0 {
                          n173 = call "CMN_toUnsc.vi"("responseQ"="dhe2unsc", "ms timeout (-1)"=5000, "command"="INIT") -> ("error out"=w515:errorcluster)  [unwired: 6 in, 2 out]
                        }
                      }
                    }
                    frame "false", "no", "off" {
                      n174 = call-poly "DatabaseHand_Set.vi"("name"="detext" ("value"), "value"=FALSE, "Database RefNum in"=w522) -> ("error out"=w520:errorcluster)  [unwired: 5 in, 3 out]
                      n175 = call "GEOM_CallGeometry.vi"("Command"="GET HEADER", "error in (no error)"=w520) -> ("error out"=w519:errorcluster)  [unwired: 13 out]
                      n176 = stacked-sequence {
                        tunnel: w519 -> [_]
                        frame #0 {
                          n177 = call "CMN_toUnsc.vi"("command"="INIT") -> ()  [unwired: 8 in, 3 out]
                        }
                      }
                    }
                  }
                }
              }
              n178 = Unbundle By Name(w485) -> ("code"=w493:i32)
            }
            frame "tempexptime" {
              # "if returned:\nvalue<0 ==> error\nvalue==0 ==> OK, value  as requested\nvalue>0 ==> it is the actual expoure time set, in ms"
              n179 = case shown="\"\", \" \", \"milliseconds\", \"millisecs\", \"ms\"" w535 {
                tunnel: [w550 w552 u32 0] -> w540
                tunnel: w532 -> [w549 w560 w568]
                tunnel: [w549 w560 w564] -> w541
                tunnel: w534 -> [w548 w559 _]
                tunnel: [w544 w556 w562] -> w538
                frame "s", "seconds", "secs" {
                  n180 = Scan From String(format string="%g", input string=w548) -> (output 1=w544:dbl)  [unwired: 2 in, 4 out]
                  n181 = Less Than 0?(x=w544) -> (x < 0?=w545:bool)
                  n182 = Select(t=0.0, s=w545, f=w544) -> (s? t:f=w543:dbl)
                  n183 = Multiply(x=w543, y=1000.0) -> (x*y=w546:dbl)
                  n184 = To Unsigned Long Integer(number=w546) -> (unsigned 32bit integer=w550:u32)
                }
                frame "", " ", "milliseconds", "millisecs", "ms" {
                  n185 = Scan From String(format string="%ld", input string=w559) -> (output 1=w553:i32)  [unwired: 2 in, 4 out]
                  n186 = Less Than 0?(x=w553) -> (x < 0?=w555:bool)
                  n187 = Select(t=0, s=w555, f=w553) -> (s? t:f=w552:i32)
                  n188 = Divide(x=w552, y=1000) -> (x/y=w556:dbl)
                }
                frame Default {
                  n189 = call "DHE_GetObsParams.vi"() -> ("DHE_OBS"=w561:T7)  [unwired: 11 out]
                  n190 = Bundle By Name(cluster=w568, "status"=TRUE, "code"=-22, "source"="SET exposuretime: Time must in secs or msecs") -> (w564:errorcluster)
                  n191 = Unbundle By Name(w561) -> ("exptime"=w562:dbl)
                }
              }
              n192 = call "DHE_set_temp_exp_time.vi"("fd"=w528, "val"=w540, "error in (no error)"=w541) -> ("fd out"=w529:i32, "return value"=w539:i32, "error out"=w537:errorcluster)  [unwired: 10 out]
              n193 = case shown="No Error" w537 {
                selector: w537 -> [w571 w583]
                tunnel: w540 -> [_ _]
                tunnel: w536 -> [w580 _]
                tunnel: w539 -> [w573 w584]
                tunnel: w538 -> [w576 _]
                tunnel: [w570 w584] -> w530
                tunnel: [w569 w583] -> w531
                frame No Error {
                  w570 = 0 ("return value")
                  n194 = Greater Than 0?(x=w573) -> (x > 0?=w572:bool)
                  n195 = call "DHE_GetMinExpTime.vi"() -> ("MinExpTime"=w579:sgl)  [unwired: 11 out]
                  n196 = Divide(x=w573, y=1000) -> (x/y=w575:dbl)
                  n197 = Select(t=w575, s=w572, f=w576) -> (s? t:f=w574:dbl)
                  n198 = Max & Min(x=w579, y=w574) -> (max(x,y)=w578:dbl)  [unwired: 1 out]
                  n199 = call-poly "DatabaseHand_Set.vi"("group"="obs", "name"="aexptime", "value"=w578, "Database RefNum in"=w580) -> ()  [unwired: 4 in, 4 out]
                  n200 = Bundle By Name(cluster=w571, "code"=w570) -> (w569:errorcluster)
                }
                frame Error {
                }
              }
              n201 = Format Into String(w538) -> (resulting string=w533:string)  [unwired: 3 in, 1 out]
            }
            frame "integration", "integtime" {
              n202 = Scan From String(format string="%g", input string=w594) -> (error out=w596:errorcluster, output 1=w595:dbl)  [unwired: 2 in, 3 out]
              n203 = case shown="Error" w596 {
                tunnel: [w600 w605] -> w586
                tunnel: w593 -> [w598 _]
                tunnel: w595 -> [w599 _]
                frame No Error {
                  n204 = case shown="\"s\", \"secs\"" w598 {
                    tunnel: w599 -> [w602 w604]
                    tunnel: [w601 w604] -> w600
                    frame Default {
                      # "def arg is in msecs"
                      n205 = Divide(x=w602, y=1000.0) -> (x/y=w601:dbl)
                    }
                    frame "s", "secs" {
                    }
                  }
                }
                frame Error {
                  n206 = call "DHE_GetObsParams.vi"() -> ("DHE_OBS"=w606:T7)  [unwired: 11 out]
                  n207 = Unbundle By Name(w606) -> ("exptime"=w605:dbl)
                }
              }
              n208 = call-poly "DatabaseHand_Set.vi"("name"="rintegtime", "value"=w586, "Database RefNum in"=w585) -> ()  [unwired: 5 in, 4 out]
              n209 = Format Into String(w586) -> (resulting string=w588:string)  [unwired: 3 in, 1 out]
            }
          }
          n210 = call "DHE_SetImageParams.vi"("DHE_IMAGE"=w33) -> ()  [unwired: 11 out]
        }
        frame "obs" {
          n211 = call "DHE_GetObsParams.vi"() -> ("DHE_OBS"=w612:T7)  [unwired: 11 out]
          n212 = case shown="\"roi\"" w610 {
            selector: w610 -> [w622 _ _ _ _ _ _ _ _ _ _ _ _ _ _ _ _ _ _ _ _ _ _ _]
            tunnel: w621 -> [_ w631 w641 w655 w665 w675 w689 w700 w708 w738 w781 w841 w852 w875 w895 w916 w949 w996 w1023 w1060 w1097 w1136 w1168 w1207]
            tunnel: [u32 22 ("code") u32 0 ("code") w643 u32 0 ("code") u32 0 ("code") u32 0 ("code") u32 0 ("code") u32 0 ("code") w712 w742 w769 w833 w855 w878 u32 0 ("code") w921 w954 w998 w1031 w1068 w1105 w1144 w1169 w1208] -> w620
            tunnel: w619 -> [w625 w637 w647 w656 w669 w679 w691 w702 w710 w740 w780 w835 w856 w877 w897 w919 w952 w1004 w1028 w1065 w1102 w1141 w1172 w1211]
            tunnel: [w624 w637 w646 w656 w669 w679 w691 w702 w710 w740 w778 w834 w856 w877 w897 w919 w952 w999 w1027 w1064 w1101 w1140 w1164 w1203] -> w618
            tunnel: w617 -> [w629 w636 w648 w658 w672 w682 w694 w705 w714 w744 w779 w836 w851 w873 w891 w922 w955 w981 w1033 w1070 w1107 w1146 w1171 w1210]
            tunnel: [w623 w636 w644 w658 w672 w682 w694 w705 w713 w743 w767 w830 w850 w872 w890 w922 w955 w982 w1032 w1069 w1106 w1145 w1170 w1209] -> w609
            tunnel: w616 -> [w627 _ _ _ _ _ _ _ _ _ _ _ _ _ _ _ _ _ _ _ _ _ _ _]
            tunnel: w615 -> [_ _ _ _ _ _ _ _ _ _ w782 _ _ _ _ _ _ _ _ _ _ _ _ _]
            tunnel: w614 -> [_ _ _ _ _ _ _ _ _ _ _ _ _ _ _ w920 w953 _ _ _ _ _ _ _]
            tunnel: w612 -> [w626 w635 w649 w657 w671 w681 w693 w704 w711 w741 w775 w840 w849 w874 w899 w918 w951 w1005 w1026 w1063 w1100 w1139 w1173 w1212]
            tunnel: [w626 w634 w645 w657 w671 w681 w693 w704 w711 w741 w776 w839 w854 w876 w899 w917 w950 w1005 w1025 w1062 w1099 w1138 w1173 w1212] -> w613
            tunnel: w611 -> [_ _ _ w659 w668 w678 w690 w701 w709 w739 w773 _ _ _ w892 _ _ _ w1024 w1061 w1098 w1137 w1166 w1205]
            tunnel: [w622 w630 w639 w655 w666 w676 w689 w700 w708 w738 w772 w831 w847 w869 w896 w915 w948 w997 w1023 w1060 w1097 w1136 w1168 w1207] -> w608
            tunnel: w607 -> [_ _ _ _ _ _ _ _ _ _ _ _ _ _ _ _ _ w993 _ _ _ _ _ _]
            frame Default {
              n213 = call "DHE_send_custom.vi"("valid params"=w627, "error in (no error)"=w629, "args"=w622, "fd"=w625) -> ("error IO"=w623:errorcluster, "fd out"=w624:i32)  [unwired: 6 out]
            }
            frame "observer" {
              n214 = Empty String/Path?(string/path=w631) -> (empty?=w633:bool)
              n215 = Select(t="unknown", s=w633, f=w631) -> (s? t:f=w630:string)
              n216 = Bundle By Name(cluster=w635, "observer"=w630) -> (w634:T7)
            }
            frame "obstype", "type" {
              n217 = call "DHE_ImtypeActions.vi"("error in (no error)"=w648, "imtype"=w641, "fd in"=w647) -> ("error out"=w644:errorcluster, "fd out"=w646:i32)  [unwired: 7 out]
              n218 = Empty String/Path?(string/path=w641) -> (empty?=w642:bool)
              n219 = Select(t="none", s=w642, f=w641) -> (s? t:f=w639:string)
              n220 = case shown="No Error" w644 {
                tunnel: w649 -> [w652 w653]
                tunnel: [w651 w653] -> w645
                tunnel: w639 -> [w650 _]
                frame No Error {
                  n221 = Bundle By Name(cluster=w652, "obstype"=w650) -> (w651:T7)
                }
                frame Error {
                }
              }
              n222 = Unbundle By Name(w644) -> ("code"=w643:i32)
            }
            frame "obsidcounter" {
              n223 = Scan From String(format string="%d", input string=w655) -> (output 1=w661:i32)  [unwired: 2 in, 4 out]
              n224 = To Unsigned Long Integer(number=w661) -> (unsigned 32bit integer=w660:u32)
              n225 = call-poly "DatabaseHand_Set.vi"("group"="obs", "name"="obsIDcounter" ("value"), "value"=w660, "Database RefNum in"=w659) -> ()  [unwired: 4 in, 4 out]
            }
            frame "obsidbase" {
              # "static"
              n226 = call "CMN_GetFromCmdLine.vi"("str in"=w665) -> ("str out"=w667:string)  [unwired: 10 out]
              n227 = call "CMN_GetFromEnv.vi"("str in"=w667) -> ("str out"=w666:string)  [unwired: 10 out]
              n228 = call-poly "DatabaseHand_Set.vi"("group"="obs", "name"="obsIDbase" ("value"), "value"=w666, "Database RefNum in"=w668) -> ()  [unwired: 4 in, 4 out]
            }
            frame "nightidbase" {
              # "static"
              n229 = call "CMN_GetFromCmdLine.vi"("str in"=w675) -> ("str out"=w677:string)  [unwired: 10 out]
              n230 = call "CMN_GetFromEnv.vi"("str in"=w677) -> ("str out"=w676:string)  [unwired: 10 out]
              n231 = call-poly "DatabaseHand_Set.vi"("group"="obs", "name"="nightIDbase" ("value"), "value"=w676, "Database RefNum in"=w678) -> ()  [unwired: 4 in, 4 out]
            }
            frame "id", "obsid" {
              w686 = "obs" ("group")
              n232 = call-poly "DatabaseHand_Set.vi"("group"=w686, "name"="obsID" ("value"), "value"=w689, "Database RefNum in"=w690) -> ("error out"=w688:errorcluster, "Database RefNum out"=w687:T1)  [unwired: 4 in, 2 out]
              n233 = call-poly "DatabaseHand_Set.vi"("group"=w686, "name"="lastobsID", "error in (no error)"=w688, "Database RefNum in"=w687) -> ()  [unwired: 4 in, 4 out]
            }
            frame "nightid" {
              w697 = "obs" ("group")
              n234 = call-poly "DatabaseHand_Set.vi"("group"=w697, "name"="nightD" ("value"), "value"=w700, "Database RefNum in"=w701) -> ("error out"=w699:errorcluster, "Database RefNum out"=w698:T1)  [unwired: 4 in, 2 out]
              n235 = call-poly "DatabaseHand_Set.vi"("group"=w697, "name"="lastnightID", "error in (no error)"=w699, "Database RefNum in"=w698) -> ()  [unwired: 4 in, 4 out]
            }
            frame "autoobsid" {
              n236 = call <vilib>:"Trim Whitespace.vi"("string"=w708) -> ("trimmed string"=w707:string)  [unwired: 1 in]
              n237 = case shown="\"on\", \"true\", \"yes\"" w707 {
                tunnel: w709 -> [_ w726 w736]
                tunnel: "autoobsID" ("value") -> [_ w724 w734]
                tunnel: w714 -> [w721 w723 w733]
                tunnel: [w720 w723 w733] -> w713
                tunnel: "obs" ("group") -> [_ _ w732]
                tunnel: [w717 0 ("code") 0 ("code")] -> w712
                frame Default {
                  w717 = -22 ("code")
                  n238 = Bundle By Name(cluster=w721, "status"=TRUE, "code"=w717, "source"="ERROR autoobsid <on | off>") -> (w720:errorcluster)
                }
                frame "on", "true", "yes" {
                  n239 = call-poly "DatabaseHand_Set.vi"("group"="obs", "name"=w724, "value"=TRUE, "Database RefNum in"=w726) -> ()  [unwired: 4 in, 4 out]
                }
                frame "", "false", "no", "off" {
                  n240 = call-poly "DatabaseHand_Set.vi"("group"=w732, "name"=w734, "value"=FALSE, "Database RefNum in"=w736) -> ("Database RefNum out"=w730:T1)  [unwired: 4 in, 3 out]
                  n241 = call-poly "DatabaseHand_Set.vi"("name"="obsID", "value"="_UNDEF_", "Database RefNum in"=w730) -> ()  [unwired: 5 in, 4 out]
                }
              }
            }
            frame "autonightid" {
              n242 = call <vilib>:"Trim Whitespace.vi"("string"=w738) -> ("trimmed string"=w737:string)  [unwired: 1 in]
              n243 = case shown="\"on\", \"true\", \"yes\"" w737 {
                tunnel: w739 -> [_ w756 w766]
                tunnel: "autonightID" ("value") -> [_ w754 w764]
                tunnel: w744 -> [w751 w753 w763]
                tunnel: [w750 w753 w763] -> w743
                tunnel: "obs" ("group") -> [_ _ w762]
                tunnel: [w747 0 ("code") 0 ("code")] -> w742
                frame Default {
                  w747 = -22 ("code")
                  n244 = Bundle By Name(cluster=w751, "status"=TRUE, "code"=w747, "source"="ERROR autoobsid <on | off>") -> (w750:errorcluster)
                }
                frame "on", "true", "yes" {
                  n245 = call-poly "DatabaseHand_Set.vi"("group"="obs", "name"=w754, "value"=TRUE, "Database RefNum in"=w756) -> ()  [unwired: 4 in, 4 out]
                }
                frame "", "false", "no", "off" {
                  n246 = call-poly "DatabaseHand_Set.vi"("group"=w762, "name"=w764, "value"=FALSE, "Database RefNum in"=w766) -> ("Database RefNum out"=w760:T1)  [unwired: 4 in, 3 out]
                  n247 = call-poly "DatabaseHand_Set.vi"("name"="nightID", "value"="_UNDEF_", "Database RefNum in"=w760) -> ()  [unwired: 5 in, 4 out]
                }
              }
            }
            frame "exposuretime", "exptime" {
              # "if returned:\nvalue<0 ==> error\nvalue==0 ==> OK, value  as requested\nvalue>0 ==> it is the actual expoure time set, in ms"
              n248 = case shown="\"\", \" \", \"milliseconds\", \"millisecs\", \"ms\"" w782 {
                tunnel: [w792 w795 u32 0] -> w777
                tunnel: w779 -> [w791 w802 w810]
                tunnel: [w791 w802 w806] -> w783
                tunnel: w781 -> [w790 w801 _]
                tunnel: [w785 w798 w803] -> w770
                tunnel: w775 -> [_ _ w804]
                frame "s", "seconds", "secs" {
                  n249 = Scan From String(format string="%g", input string=w790) -> (output 1=w785:dbl)  [unwired: 2 in, 4 out]
                  n250 = Less Than 0?(x=w785) -> (x < 0?=w787:bool)
                  n251 = Select(t=0.0, s=w787, f=w785) -> (s? t:f=w784:dbl)
                  n252 = Multiply(x=w784, y=1000.0) -> (x*y=w788:dbl)
                  n253 = To Unsigned Long Integer(number=w788) -> (unsigned 32bit integer=w792:u32)
                }
                frame "", " ", "milliseconds", "millisecs", "ms" {
                  n254 = Scan From String(format string="%ld", input string=w801) -> (output 1=w796:i32)  [unwired: 2 in, 4 out]
                  n255 = Less Than 0?(x=w796) -> (x < 0?=w797:bool)
                  n256 = Select(t=0, s=w797, f=w796) -> (s? t:f=w795:i32)
                  n257 = Divide(x=w795, y=1000) -> (x/y=w798:dbl)
                }
                frame Default {
                  n258 = Unbundle By Name(w804) -> ("exptime"=w803:dbl)
                  n259 = Bundle By Name(cluster=w810, "status"=TRUE, "code"=-22, "source"="SET exposuretime: Time must in secs or msecs") -> (w806:errorcluster)
                }
              }
              n260 = call "DHE_set_exp_time.vi"("fd"=w780, "val"=w777, "error in (no error)"=w783) -> ("fd out"=w778:i32, "return value"=w771:i32, "error out"=w768:errorcluster)  [unwired: 10 out]
              n261 = Unbundle By Name(w775) -> ("exptime"=w774:dbl)
              n262 = case shown="No Error" w768 {
                selector: w768 -> [w813 w827]
                tunnel: w777 -> [_ _]
                tunnel: w775 -> [w826 w829]
                tunnel: [w825 w829] -> w776
                tunnel: w774 -> [_ _]
                tunnel: w773 -> [w822 _]
                tunnel: w771 -> [w815 w828]
                tunnel: w770 -> [w818 _]
                tunnel: [w812 w828] -> w769
                tunnel: [w811 w827] -> w767
                frame No Error {
                  w812 = 0 ("return value")
                  n263 = Greater Than 0?(x=w815) -> (x > 0?=w814:bool)
                  n264 = call "DHE_GetMinExpTime.vi"() -> ("MinExpTime"=w821:sgl)  [unwired: 11 out]
                  n265 = Divide(x=w815, y=1000) -> (x/y=w817:dbl)
                  n266 = Select(t=w817, s=w814, f=w818) -> (s? t:f=w816:dbl)
                  n267 = Max & Min(x=w821, y=w816) -> (max(x,y)=w820:dbl)  [unwired: 1 out]
                  n268 = Bundle By Name(cluster=w826, "exptime"=w820) -> (w825:T7)
                  n269 = call-poly "DatabaseHand_Set.vi"("group"="obs", "name"="aexptime", "value"=w820, "Database RefNum in"=w822) -> ()  [unwired: 4 in, 4 out]
                  n270 = Bundle By Name(cluster=w813, "code"=w812) -> (w811:errorcluster)
                }
                frame Error {
                }
              }
              n271 = Format Into String(w770) -> (resulting string=w772:string)  [unwired: 3 in, 1 out]
            }
            frame "imagestoread", "nimages", "numreads" {
              n272 = Decimal String To Number(string=w841) -> (number=w832:i32)  [unwired: 3 out]
              n273 = Max & Min(x=w832, y=1) -> (max(x,y)=w837:i32)  [unwired: 1 out]
              n274 = call "DHE_set_nimages.vi"("fd"=w835, "val"=w837, "error in (no error)"=w836) -> ("fd out"=w834:i32, "return value"=w833:i32, "error out"=w830:errorcluster)  [unwired: 10 out]
              n275 = case shown="No Error" w830 {
                tunnel: w840 -> [w844 w845]
                tunnel: [w843 w845] -> w839
                tunnel: w832 -> [w842 _]
                frame No Error {
                  n276 = Bundle By Name(cluster=w844, "nimages"=w842) -> (w843:T7)
                }
                frame Error {
                }
              }
              n277 = Format Into String(w832) -> (resulting string=w831:string)  [unwired: 3 in, 1 out]
            }
            frame "display", "display_image", "displayimage" {
              n278 = call <vilib>:"Trim Whitespace.vi"("string"=w852) -> ("trimmed string"=w848:string)  [unwired: 1 in]
              n279 = To Lower Case(string=w848) -> (all lower case string=w846:string)
              n280 = case shown="\"false\", \"no\", \"off\"" w846 {
                tunnel: [w862 TRUE FALSE] -> w853
                tunnel: w851 -> [w860 w864 w866]
                tunnel: [w861 w864 w866] -> w850
                tunnel: w849 -> [w863 _ _]
                frame Default {
                  n281 = Unbundle By Name(w863) -> ("display"=w862:bool)
                  n282 = Bundle By Name(cluster=w860, "status"=TRUE, "code"=-22, "source"="ERROR <yes | no>") -> (w861:errorcluster)
                }
                frame "on", "true", "yes" {
                }
                frame "false", "no", "off" {
                }
              }
              n283 = Bundle By Name(cluster=w849, "display"=w853) -> (w854:T7)
              n284 = Unbundle By Name(w850) -> ("code"=w855:i32)
              n285 = Format Into String(w848) -> (resulting string=w847:string)  [unwired: 3 in, 1 out]
            }
            frame "autowrit", "write", "write_to_disk" {
              n286 = call <vilib>:"Trim Whitespace.vi"("string"=w875) -> ("trimmed string"=w870:string)  [unwired: 1 in]
              n287 = To Lower Case(string=w870) -> (all lower case string=w868:string)
              n288 = case shown="Default" w868 {
                tunnel: [w884 TRUE FALSE] -> w871
                tunnel: w873 -> [w882 w886 w888]
                tunnel: [w883 w886 w888] -> w872
                tunnel: w874 -> [w885 _ _]
                frame Default {
                  n289 = Unbundle By Name(w885) -> ("autowrite"=w884:bool)
                  n290 = Bundle By Name(cluster=w882, "status"=TRUE, "code"=-22, "source"="ERROR <yes | no>") -> (w883:errorcluster)
                }
                frame "on", "true", "yes" {
                }
                frame "false", "no", "off" {
                }
              }
              n291 = Bundle By Name(cluster=w874, "autowrite"=w871) -> (w876:T7)
              n292 = Format Into String(w868) -> (resulting string=w869:string)  [unwired: 3 in, 1 out]
              n293 = Unbundle By Name(w872) -> ("code"=w878:i32)
            }
            frame "checkdisk", "chkdisk" {
              n294 = call <vilib>:"Trim Whitespace.vi"("string"=w895) -> ("trimmed string"=w894:string)  [unwired: 1 in]
              n295 = To Lower Case(string=w894) -> (all lower case string=w893:string)
              n296 = case shown="Default" w893 {
                tunnel: w892 -> [_ w909 w914]
                tunnel: w891 -> [w904 w905 w910]
                tunnel: [w903 w905 w910] -> w890
                frame Default {
                  n297 = Bundle By Name(cluster=w904, "status"=TRUE, "code"=-22, "source"="ERROR chkdisk <on | off>") -> (w903:errorcluster)
                }
                frame "1", "on", "true", "yes" {
                  n298 = call-poly "DatabaseHand_Set.vi"("group"="obs", "name"="chkdisk", "value"=TRUE, "Database RefNum in"=w909) -> ()  [unwired: 4 in, 4 out]
                }
                frame "0", "false", "no", "off" {
                  n299 = call-poly "DatabaseHand_Set.vi"("group"="obs", "name"="chkdisk", "value"=FALSE, "Database RefNum in"=w914) -> ()  [unwired: 4 in, 4 out]
                }
              }
              n300 = Format Into String(w894) -> (resulting string=w896:string)  [unwired: 3 in, 1 out]
            }
            frame "writeframes" {
              n301 = stacked-sequence {
                seq-local: [w924 _] -> [_ w927]
                tunnel: w916 -> [_ w928]
                tunnel: w920 -> [_ _]
                tunnel: [_ w926] -> w917
                tunnel: w918 -> [w923 _]
                frame #0 {
                  w925 = FALSE
                  n302 = Bundle By Name(cluster=w923, "frames to write.subs"=w925, "frames to write.reset"=w925, "frames to write.exposed"=w925) -> (w924:T7)
                }
                frame #1 {
                  n303 = while {
                    shift-left: w927 -> [w930]
                    shift-right: [w929] -> w926
                    shift-left: w928 -> [w932]
                    shift-right: [w931] -> _
                    stop <- w936 stop-if-true
                    n304 = Scan From String(format string="%s" ("Format String"), input string=w932) -> (remaining string=w931:string, output 1=w935:string)  [unwired: 2 in, 3 out]
                    n305 = Empty String/Path?(string/path=w935) -> (empty?=w936:bool)
                    n306 = To Lower Case(string=w935) -> (all lower case string=w934:string)
                    n307 = case shown="\"exposed\"" w934 {
                      tunnel: TRUE -> [_ w939 w942 w945]
                      tunnel: w930 -> [w938 w941 w944 w947]
                      tunnel: [w938 w940 w943 w946] -> w929
                      frame Default {
                      }
                      frame "reset" {
                        n308 = Bundle By Name(cluster=w941, "frames to write.reset"=w939) -> (w940:T7)
                      }
                      frame "substracted" {
                        n309 = Bundle By Name(cluster=w944, "frames to write.subs"=w942) -> (w943:T7)
                      }
                      frame "exposed" {
                        n310 = Bundle By Name(cluster=w947, "frames to write.exposed"=w945) -> (w946:T7)
                      }
                    }
                  }
                }
              }
              n311 = Unbundle By Name(w922) -> ("code"=w921:i32)
              n312 = Format Into String(w916) -> (resulting string=w915:string)  [unwired: 3 in, 1 out]
            }
            frame "dispframes" {
              n313 = stacked-sequence {
                seq-local: [w957 _] -> [_ w960]
                tunnel: w949 -> [_ w961]
                tunnel: w953 -> [_ _]
                tunnel: [_ w959] -> w950
                tunnel: w951 -> [w956 _]
                frame #0 {
                  w958 = FALSE
                  n314 = Bundle By Name(cluster=w956, "frames to display.subs"=w958, "frames to display.reset"=w958, "frames to display.exposed"=w958) -> (w957:T7)
                }
                frame #1 {
                  n315 = while {
                    shift-left: w960 -> [w963]
                    shift-right: [w962] -> w959
                    shift-left: w961 -> [w965]
                    shift-right: [w964] -> _
                    stop <- w969 stop-if-true
                    n316 = Scan From String(format string="%s" ("Format String"), input string=w965) -> (remaining string=w964:string, output 1=w968:string)  [unwired: 2 in, 3 out]
                    n317 = Empty String/Path?(string/path=w968) -> (empty?=w969:bool)
                    n318 = To Lower Case(string=w968) -> (all lower case string=w967:string)
                    n319 = case shown="\"exposed\"" w967 {
                      tunnel: TRUE -> [_ w972 w975 w978]
                      tunnel: w963 -> [w971 w974 w977 w980]
                      tunnel: [w971 w973 w976 w979] -> w962
                      frame Default {
                      }
                      frame "reset" {
                        n320 = Bundle By Name(cluster=w974, "frames to display.reset"=w972) -> (w973:T7)
                      }
                      frame "subs", "substracted" {
                        n321 = Bundle By Name(cluster=w977, "frames to display.subs"=w975) -> (w976:T7)
                      }
                      frame "exposed" {
                        n322 = Bundle By Name(cluster=w980, "frames to display.exposed"=w978) -> (w979:T7)
                      }
                    }
                  }
                }
              }
              n323 = Unbundle By Name(w955) -> ("code"=w954:i32)
              n324 = Format Into String(w949) -> (resulting string=w948:string)  [unwired: 3 in, 1 out]
            }
            frame "roi" {
              # "xstart ystart xsize ysize"
              n325 = call "DHE_set_roi_transf.vi"("error in (no error)"=w981, "args"=w996) -> ("error out"=w994:errorcluster, "full"=w990:bool, "roi"=w995:string, "add roi"=w983:bool)  [unwired: 6 out]
              n326 = Search 1D Array(1D array=w993, element="-full") -> (index of element=w991:i32)  [unwired: 1 out]
              n327 = Greater Or Equal To 0?(x=w991) -> (x >= 0?=w989:bool)
              n328 = Scan From String(format string="%d %d %d %d" ("Format String"), input string=w995, error in=w994) -> (error out=w988:errorcluster, output 1=w1003:i32, output 2=w1002:i32, output 3=w1001:i32, output 4=w1000:i32)  [unwired: 1 in, 6 out]
              n329 = Unbundle By Name(w988) -> ("status"=w987:bool)
              n330 = Or(x=w990, y=w989) -> (x .or. y?=w985:bool)
              n331 = Not(x=w985) -> (.not. x?=w984:bool)
              n332 = And(x=w987, y=w984) -> (x .and. y?=w986:bool)
              n333 = case shown="False" w986 {
                tunnel: [w1017 w1022] -> w982
                tunnel: w1004 -> [w1016 w1020]
                tunnel: w1003 -> [w1015 _]
                tunnel: w1002 -> [w1014 _]
                tunnel: w1001 -> [w1013 _]
                tunnel: w1000 -> [w1012 _]
                tunnel: [w1011 w1020] -> w999
                tunnel: [w1010 w1019] -> w998
                tunnel: w985 -> [w1009 _]
                tunnel: w981 -> [w1008 w1018]
                tunnel: w983 -> [w1007 _]
                frame False {
                  n334 = call "DHE_SetROI.vi"("refnum"=w1016, "xsize"=w1013, "ysize"=w1012, "xstart"=w1015, "ystart"=w1014, "error in (no error)"=w1008, "new roi"=w1007, "full roi"=w1009) -> ("fd out"=w1011:i32, "return value"=w1010:i32, "error out"=w1017:errorcluster)  [unwired: 5 out]
                }
                frame True {
                  w1019 = -22 ("code")
                  n335 = Bundle By Name(cluster=w1018, "code"=w1019, "source"="ERR: roi <xstart> <ystart> <xlen> <ylen> ") -> (w1022:errorcluster)
                }
              }
              n336 = Format Into String(w995) -> (resulting string=w997:string)  [unwired: 3 in, 1 out]
            }
            frame "coadds" {
              n337 = Scan From String(format string="%d", input string=w1023) -> (error out=w1030:errorcluster, output 1=w1029:i32)  [unwired: 2 in, 3 out]
              n338 = case shown="No Error" w1030 {
                tunnel: w1033 -> [w1041 w1049]
                tunnel: [w1040 w1047] -> w1032
                tunnel: [w1037 w1048] -> w1031
                tunnel: w1029 -> [_ w1045]
                tunnel: w1028 -> [w1036 w1050]
                tunnel: [w1036 w1044] -> w1027
                tunnel: w1026 -> [w1035 w1046]
                tunnel: [w1035 w1042] -> w1025
                tunnel: w1024 -> [_ w1043]
                frame Error {
                  w1037 = -22 ("code")
                  n339 = Bundle By Name(cluster=w1041, "status"=TRUE, "code"=w1037, "source"="ERROR must be an integer number") -> (w1040:errorcluster)
                }
                frame No Error {
                  n340 = call "DHE_set_ncoadds.vi"("fd"=w1050, "val"=w1045, "error in (no error)"=w1049) -> ("fd out"=w1044:i32, "return value"=w1048:i32, "error out"=w1047:errorcluster)  [unwired: 10 out]
                  n341 = case shown="No Error" w1047 {
                    selector: w1047 -> [w1055 w1058]
                    tunnel: w1045 -> [w1053 _]
                    tunnel: w1046 -> [w1057 w1059]
                    tunnel: [w1052 w1059] -> w1042
                    tunnel: w1044 -> [w1051 _]
                    tunnel: w1043 -> [w1056 _]
                    tunnel: [w1054 w1058] -> _
                    frame No Error {
                      n342 = Bundle By Name(cluster=w1057, "coadds"=w1053) -> (w1052:T7)
                      n343 = call "DHE_autoSample.vi"("error in"=w1055, "fd"=w1051, "DHE_OBS"=w1052, "DBSRef"=w1056) -> ("error out"=w1054:errorcluster)  [unwired: 3 in, 4 out]
                    }
                    frame Error {
                    }
                  }
                }
              }
            }
            frame "sur" {
              n344 = Scan From String(format string="%d", input string=w1060) -> (error out=w1067:errorcluster, output 1=w1066:i32)  [unwired: 2 in, 3 out]
              n345 = case shown="No Error" w1067 {
                tunnel: w1070 -> [w1078 w1087]
                tunnel: [w1077 w1085] -> w1069
                tunnel: [w1074 w1086] -> w1068
                tunnel: w1066 -> [_ w1082]
                tunnel: w1065 -> [w1073 w1083]
                tunnel: [w1073 w1081] -> w1064
                tunnel: w1063 -> [w1072 w1084]
                tunnel: [w1072 w1079] -> w1062
                tunnel: w1061 -> [_ w1080]
                frame Error {
                  w1074 = -22 ("code")
                  n346 = Bundle By Name(cluster=w1078, "status"=TRUE, "code"=w1074, "source"="ERROR must be an integer number") -> (w1077:errorcluster)
                }
                frame No Error {
                  n347 = call "DHE_set_nsur.vi"("fd"=w1083, "val"=w1082, "error in (no error)"=w1087) -> ("fd out"=w1081:i32, "return value"=w1086:i32, "error out"=w1085:errorcluster)  [unwired: 10 out]
                  n348 = case shown="No Error" w1085 {
                    selector: w1085 -> [w1092 w1095]
                    tunnel: w1082 -> [w1090 _]
                    tunnel: w1084 -> [w1094 w1096]
                    tunnel: [w1088 w1096] -> w1079
                    tunnel: w1081 -> [w1089 _]
                    tunnel: w1080 -> [w1093 _]
                    tunnel: [w1091 w1095] -> _
                    frame No Error {
                      n349 = Bundle By Name(cluster=w1094, "sur"=w1090) -> (w1088:T7)
                      n350 = call "DHE_autoSample.vi"("error in"=w1092, "fd"=w1089, "DHE_OBS"=w1088, "DBSRef"=w1093) -> ("error out"=w1091:errorcluster)  [unwired: 3 in, 4 out]
                    }
                    frame Error {
                    }
                  }
                }
              }
            }
            frame "fowler", "fsample" {
              n351 = Scan From String(format string="%d", input string=w1097) -> (error out=w1104:errorcluster, output 1=w1103:i32)  [unwired: 2 in, 3 out]
              n352 = case shown="No Error" w1104 {
                tunnel: w1107 -> [w1115 w1124]
                tunnel: [w1114 w1116] -> w1106
                tunnel: [w1111 w1123] -> w1105
                tunnel: w1103 -> [_ w1122]
                tunnel: w1102 -> [w1110 w1125]
                tunnel: [w1110 w1118] -> w1101
                tunnel: w1100 -> [w1109 w1120]
                tunnel: [w1109 w1119] -> w1099
                tunnel: w1098 -> [_ w1117]
                frame Error {
                  w1111 = -22 ("code")
                  n353 = Bundle By Name(cluster=w1115, "status"=TRUE, "code"=w1111, "source"="ERROR must be an integer number") -> (w1114:errorcluster)
                }
                frame No Error {
                  n354 = call "DHE_set_fsamples.vi"("fd"=w1125, "val"=w1122, "error in (no error)"=w1124) -> ("fd out"=w1118:i32, "return value"=w1123:i32, "error out"=w1121:errorcluster)  [unwired: 10 out]
                  n355 = case shown="No Error" w1121 {
                    selector: w1121 -> [w1131 w1134]
                    tunnel: w1122 -> [w1129 _]
                    tunnel: w1120 -> [w1133 w1135]
                    tunnel: [w1128 w1135] -> w1119
                    tunnel: w1118 -> [w1127 _]
                    tunnel: w1117 -> [w1132 _]
                    tunnel: [w1130 w1134] -> w1116
                    frame No Error {
                      n356 = Bundle By Name(cluster=w1133, "fowler"=w1129) -> (w1128:T7)
                      n357 = call "DHE_autoSample.vi"("autoampling"=TRUE, "error in"=w1131, "fd"=w1127, "DHE_OBS"=w1128, "DBSRef"=w1132) -> ("error out"=w1130:errorcluster)  [unwired: 2 in, 4 out]
                    }
                    frame Error {
                    }
                  }
                }
              }
            }
            frame "nsample", "nsamples" {
              n358 = Scan From String(format string="%d", input string=w1136) -> (error out=w1143:errorcluster, output 1=w1142:i32)  [unwired: 2 in, 3 out]
              n359 = case shown="No Error" w1143 {
                tunnel: w1146 -> [w1154 w1158]
                tunnel: [w1153 w1157] -> w1145
                tunnel: [w1150 w1161] -> w1144
                tunnel: w1142 -> [_ w1159]
                tunnel: w1141 -> [w1149 w1163]
                tunnel: [w1149 w1162] -> w1140
                tunnel: w1139 -> [w1148 _]
                tunnel: [w1148 w1160] -> w1138
                tunnel: w1137 -> [_ w1156]
                frame Error {
                  w1150 = -22 ("code")
                  n360 = Bundle By Name(cluster=w1154, "status"=TRUE, "code"=w1150, "source"="ERROR must be an integer number") -> (w1153:errorcluster)
                }
                frame No Error {
                  n361 = call "DHE_SetNPixSamples.vi"("Database RefNum in"=w1156, "error in (no error)"=w1158, "check sampling"=TRUE, "nsamples"=w1159, "fd"=w1163) -> ("error IO"=w1157:errorcluster, "DHE_OBS"=w1160:T7, "return value"=w1161:i32, "fd out"=w1162:i32)  [unwired: 3 out]
                }
              }
            }
            frame "seqdelay" {
              n362 = Scan From String(format string="%g", input string=w1168) -> (output 1=w1165:dbl)  [unwired: 2 in, 4 out]
              n363 = call "DHE_set_seqdelay.vi"("fd"=w1172, "val"=w1165, "error in (no error)"=w1171) -> ("fd out"=w1164:i32, "return value"=w1169:i32, "error out"=w1170:errorcluster)  [unwired: 10 out]
              n364 = case shown="No Error" w1170 {
                tunnel: w1166 -> [w1175 _]
                tunnel: w1165 -> [w1176 _]
                tunnel: w1164 -> [w1174 _]
                frame No Error {
                  # "recalc readtime"
                  n365 = stacked-sequence {
                    tunnel: w1176 -> [w1179 _]
                    tunnel: w1175 -> [w1181 w1186]
                    tunnel: w1174 -> [w1180 _]
                    frame #0 {
                      n366 = call "DHE_get_intdelay.vi"("fd in"=w1180) -> ("msdelay"=w1178:sgl)  [unwired: 1 in, 13 out]
                      n367 = Add(x=w1179, y=w1178) -> (x+y=w1177:dbl)
                      n368 = call "DHE_GetTimingInfo.vi"("Database RefNum out"=w1181) -> ("Timing"=w1184:T8)  [unwired: 10 out]
                      n369 = Divide(x=w1177, y=1000.0) -> (x/y=w1183:dbl)
                      n370 = Bundle By Name(cluster=w1184, "known_overhead"=w1183) -> (w1185:T8)
                      n371 = call "DHE_SetTimingInfo.vi"("Timing"=w1185, "Database RefNum out"=w1181) -> ()  [unwired: 10 out]
                    }
                    frame #1 {
                      n372 = call "DHE_GetReadMode.vi"() -> ("DHE_ReadMode"=w1189:string)  [unwired: 9 out]
                      n373 = call "DHE_GetDetXYSize.vi"() -> ("DHE_DetYsize"=w1188:i32, "DHE_DetXsize"=w1187:i32)  [unwired: 8 out]
                      n374 = call "GEOM_GetFPA.vi"("readmode"=w1189) -> ("CorrectedFPACoord"=w1190:T9, "amplifiers"=w1197:T10[], "numyamps"=w1194:i32, "numxamps"=w1195:i32)  [unwired: 2 in, 5 out]
                      n375 = Unbundle By Name(w1190) -> ("totxsize"=w1191:i32, "totysize"=w1192:i32)
                      n376 = Index Array(array=w1197, index=0) -> (element=w1198:T10)
                      n377 = Array Size(array=w1197) -> (size(s)=w1193:i32)
                      n378 = Unbundle By Name(w1198) -> ("Corr ROI"=w1199:T12)
                      n379 = Index Array(array=w1199, index=0) -> (element=w1201:T13)
                      n380 = Unbundle By Name(w1201) -> ("ystart"=w1202:u32)
                      n381 = call "DHE_SetTiming.vi"("num of Y amps"=w1194, "num of X amps"=w1195, "yroi start"=w1202, "roi rows"=w1192, "Num of amps"=w1193, "roi cols"=w1191, "totysize"=w1188, "totxsize"=w1187, "Database RefNum out"=w1186) -> ()  [unwired: 1 in, 2 out]
                    }
                  }
                }
                frame Error {
                }
              }
            }
            frame "intdelay" {
              n382 = Scan From String(format string="%g", input string=w1207) -> (output 1=w1204:dbl)  [unwired: 2 in, 4 out]
              n383 = call "DHE_set_intdelay.vi"("fd"=w1211, "val"=w1204, "error in (no error)"=w1210) -> ("fd out"=w1203:i32, "return value"=w1208:i32, "error out"=w1209:errorcluster)  [unwired: 10 out]
              n384 = case shown="No Error" w1209 {
                tunnel: w1205 -> [w1214 _]
                tunnel: w1204 -> [w1215 _]
                tunnel: w1203 -> [w1213 _]
                frame No Error {
                  # "recalc readtime"
                  n385 = stacked-sequence {
                    tunnel: w1215 -> [w1218 _]
                    tunnel: w1214 -> [w1220 w1225]
                    tunnel: w1213 -> [w1219 _]
                    frame #0 {
                      n386 = call "DHE_get_seqdelay.vi"("fd in"=w1219) -> ("idle"=w1217:sgl)  [unwired: 1 in, 13 out]
                      n387 = Add(x=w1218, y=w1217) -> (x+y=w1216:dbl)
                      n388 = call "DHE_GetTimingInfo.vi"("Database RefNum out"=w1220) -> ("Timing"=w1223:T8)  [unwired: 10 out]
                      n389 = Divide(x=w1216, y=1000.0) -> (x/y=w1222:dbl)
                      n390 = Bundle By Name(cluster=w1223, "known_overhead"=w1222) -> (w1224:T8)
                      n391 = call "DHE_SetTimingInfo.vi"("Timing"=w1224, "Database RefNum out"=w1220) -> ()  [unwired: 10 out]
                    }
                    frame #1 {
                      n392 = call "DHE_GetReadMode.vi"() -> ("DHE_ReadMode"=w1228:string)  [unwired: 9 out]
                      n393 = call "DHE_GetDetXYSize.vi"() -> ("DHE_DetYsize"=w1227:i32, "DHE_DetXsize"=w1226:i32)  [unwired: 8 out]
                      n394 = call "GEOM_GetFPA.vi"("readmode"=w1228) -> ("CorrectedFPACoord"=w1229:T9, "amplifiers"=w1236:T10[], "numyamps"=w1233:i32, "numxamps"=w1234:i32)  [unwired: 2 in, 5 out]
                      n395 = Unbundle By Name(w1229) -> ("totxsize"=w1230:i32, "totysize"=w1231:i32)
                      n396 = Index Array(array=w1236, index=0) -> (element=w1237:T10)
                      n397 = Array Size(array=w1236) -> (size(s)=w1232:i32)
                      n398 = Unbundle By Name(w1237) -> ("Corr ROI"=w1238:T12)
                      n399 = Index Array(array=w1238, index=0) -> (element=w1240:T13)
                      n400 = Unbundle By Name(w1240) -> ("ystart"=w1241:u32)
                      n401 = call "DHE_SetTiming.vi"("num of Y amps"=w1233, "num of X amps"=w1234, "yroi start"=w1241, "roi rows"=w1231, "Num of amps"=w1232, "roi cols"=w1230, "totysize"=w1227, "totxsize"=w1226, "Database RefNum out"=w1225) -> ()  [unwired: 1 in, 2 out]
                    }
                  }
                }
                frame Error {
                }
              }
            }
          }
          n402 = call "DHE_SetObsParams.vi"("DHE_OBS"=w613) -> ()  [unwired: 11 out]
        }
        frame "dhe" {
          n403 = case shown="\"deftiming\", \"timing\"" w1246 {
            selector: w1246 -> [w1256 _ _ _ _ _ _ _ _ _ _ _ _ _ _ w1547 _ _ _ _ _ _]
            tunnel: w1252 -> [w1262 w1269 w1307 w1314 w1330 w1353 w1388 w1430 w1439 w1453 w1485 w1503 w1509 w1520 w1538 w1557 w1604 w1690 w1701 w1721 w1746 w1796]
            tunnel: w1251 -> [w1259 w1266 w1306 w1316 w1336 w1357 w1383 w1429 w1437 w1455 w1483 w1499 w1508 w1521 w1539 w1558 w1607 w1691 w1705 w1725 w1748 w1793]
            tunnel: [w1258 w1265 w1301 w1315 w1335 w1356 w1389 w1428 w1436 w1455 w1482 w1500 w1507 w1516 w1534 w1553 w1607 w1686 w1705 w1725 w1747 w1793] -> w1250
            tunnel: [0 ("return value") w1267 w1304 w1312 w1333 w1355 w1390 w1426 w1434 0 ("code") w1480 w1501 w1506 w1515 w1533 w1552 w1602 w1685 w1699 w1719 w1744 w1794] -> w1249
            tunnel: [w1257 w1264 w1302 w1313 w1334 w1354 w1387 w1427 w1435 w1452 w1481 w1502 w1505 w1519 w1537 w1556 w1603 w1689 w1700 w1720 w1745 w1795] -> w1248
            tunnel: w1247 -> [w1253 w1271 w1298 w1311 w1337 w1358 w1376 w1425 w1438 w1458 w1484 w1497 w1504 w1522 w1531 w1550 w1613 w1683 w1698 w1718 w1738 _]
            tunnel: w1244 -> [_ _ _ _ _ _ _ _ _ _ _ _ _ _ _ _ _ _ _ _ _ _]
            tunnel: w1245 -> [w1260 _ _ _ _ _ _ _ _ _ _ _ _ _ _ _ _ _ _ _ _ _]
            tunnel: w1244 -> [_ w1270 _ _ _ _ _ _ _ _ _ _ _ w1517 w1535 w1554 w1614 w1687 _ _ w1743 _]
            tunnel: w1243 -> [_ _ _ _ _ _ w1386 _ _ w1456 w1476 w1498 _ _ _ w1548 w1608 w1681 _ _ w1739 _]
            tunnel: [w1253 w1263 w1298 w1311 w1337 w1351 w1378 w1425 w1431 w1457 w1477 w1497 w1504 w1513 w1532 w1549 w1612 w1682 w1697 w1717 w1737 "" ("trimmed string")] -> w1242
            frame Default {
              n404 = Concatenate Strings(w1256, " " ("string"), w1253) -> (w1255:string)
              n405 = call "DHE_send_custom.vi"("valid params"=w1260, "error in (no error)"=w1262, "args"=w1255, "fd"=w1259) -> ("error IO"=w1257:errorcluster, "fd out"=w1258:i32)  [unwired: 6 out]
            }
            frame "idle", "idlemode" {
              n406 = Scan From String(format string="%s" ("Format String"), input string=w1271) -> (output 1=w1263:string)  [unwired: 2 in, 4 out]
              n407 = To Lower Case(string=w1263) -> (all lower case string=w1272:string)
              n408 = case shown="\"on\", \"start\", \"yes\"" w1272 {
                tunnel: w1269 -> [w1277 w1286 w1293]
                tunnel: [w1276 w1285 w1289] -> w1264
                tunnel: [TRUE FALSE FALSE] -> w1268
                tunnel: [w1278 w1282 w1290] -> w1267
                tunnel: w1266 -> [w1280 w1283 w1292]
                tunnel: [w1279 w1283 w1291] -> w1265
                frame "on", "start", "yes" {
                  (unwired) TRUE
                  n409 = call "DHE_idle.vi"("fd"=w1280, "flag"=i8 1, "error in (no error)"=w1277) -> ("fd out"=w1279:i32, "return value"=w1278:i32, "error out"=w1276:errorcluster)  [unwired: 10 out]
                }
                frame Default {
                  w1282 = -22 ("code")
                  (unwired) FALSE
                  n410 = Bundle By Name(cluster=w1286, "source"="unknow parameter", "code"=w1282, "status"=TRUE) -> (w1285:errorcluster)
                }
                frame "false", "no", "off", "stop" {
                  n411 = call "DHE_idle.vi"("fd"=w1292, "flag"=i8 0, "error in (no error)"=w1293) -> ("fd out"=w1291:i32, "return value"=w1290:i32, "error out"=w1289:errorcluster)  [unwired: 10 out]
                }
              }
              n412 = case shown="No Error" w1264 {
                tunnel: w1270 -> [w1296 _]
                tunnel: w1268 -> [w1295 _]
                frame No Error {
                  n413 = Bundle By Name(cluster=w1296, "idlemode"=w1295) -> (w1297:T5)
                  n414 = call "DHE_SetControllerParams.vi"("ControllerStatus"=w1297) -> ()  [unwired: 1 in, 10 out]
                }
                frame Error {
                }
              }
            }
            frame "readmode", "readoutmode" {
              n415 = call "GEOM_GetModifiers.vi"() -> ("GEOM_modifiers"=w1305:T14)  [unwired: 1 in, 10 out]
              n416 = Unbundle By Name(w1305) -> ("Binning.x"=w1300:u32, "Binning.y"=w1299:u32)
              n417 = call "DHE_SetReadMode.vi"("refnum"=w1306, "readmode"=w1298, "error in (no error)"=w1307) -> ("fd out"=w1301:i32, "error out"=w1303:errorcluster)  [unwired: 11 out]
              n418 = call "DHE_SetBinning.vi"("refnum"=w1301, "xbin"=w1300, "ybin"=w1299, "error in (no error)"=w1303) -> ("return value"=w1304:i32, "error out"=w1302:errorcluster)  [unwired: 10 out]
            }
            frame "binning" {
              n419 = call "DHE_ParseBinning.vi"("binning"=w1311) -> ("error out"=w1310:errorcluster, "ybining"=w1308:i32, "xbining"=w1309:i32)  [unwired: 1 in, 7 out]
              n420 = case shown="No Error" w1310 {
                tunnel: w1308 -> [w1323 _]
                tunnel: w1309 -> [w1322 _]
                tunnel: w1316 -> [w1321 w1329]
                tunnel: [w1320 w1329] -> w1315
                tunnel: w1314 -> [w1319 w1326]
                tunnel: [w1318 w1325] -> w1313
                tunnel: [w1317 w1324] -> w1312
                frame No Error {
                  n421 = call "DHE_SetBinning.vi"("refnum"=w1321, "xbin"=w1322, "ybin"=w1323, "error in (no error)"=w1319) -> ("fd out"=w1320:i32, "return value"=w1317:i32, "error out"=w1318:errorcluster)  [unwired: 9 out]
                }
                frame Error {
                  w1324 = -22 ("code")
                  n422 = Bundle By Name(cluster=w1326, "status"=TRUE, "code"=w1324, "source"="ERROR: binning <xbin> <ybin>") -> (w1325:errorcluster)
                }
              }
            }
            frame "bpp" {
              n423 = Scan From String(format string="%d", input string=w1337) -> (error out=w1331:errorcluster, output 1=w1332:i32)  [unwired: 2 in, 3 out]
              n424 = case shown="No Error" w1331 {
                tunnel: w1336 -> [w1344 w1350]
                tunnel: [w1343 w1350] -> w1335
                tunnel: [w1342 w1348] -> w1334
                tunnel: [w1341 w1345] -> w1333
                tunnel: w1332 -> [w1340 _]
                tunnel: w1330 -> [w1339 w1349]
                frame No Error {
                  n425 = call "DHE_ChangeRawBpp.vi"("error in (no error)"=w1339, "bpp"=w1340, "fd"=w1344) -> ("error out"=w1342:errorcluster, "fd out"=w1343:i32)  [unwired: 7 out]
                  n426 = Unbundle By Name(w1342) -> ("code"=w1341:i32)
                }
                frame Error {
                  w1345 = -22 ("code")
                  n427 = Bundle By Name(cluster=w1349, "status"=TRUE, "code"=w1345, "source"="ERROR bpp must be an integer number") -> (w1348:errorcluster)
                }
              }
            }
            frame "artifdata" {
              n428 = Scan From String(format string="%s" ("Format String"), input string=w1358) -> (output 1=w1352:string)  [unwired: 2 in, 4 out]
              n429 = To Lower Case(string=w1352) -> (all lower case string=w1351:string)
              n430 = case shown="Default" w1351 {
                selector: w1351 -> [w1365 _ _]
                tunnel: [w1364 1 0] -> w1359
                tunnel: [w1363 TRUE FALSE] -> w1360
                frame Default {
                  n431 = Decimal String To Number(string=w1365) -> (number=w1364:i32)  [unwired: 3 out]
                  n432 = Not Equal To 0?(x=w1364) -> (x != 0?=w1363:bool)
                }
                frame "on", "true", "yes" {
                }
                frame "false", "no", "off" {
                }
              }
              n433 = call "DHE_artif_data.vi"("fd"=w1357, "flag"=w1359, "error in (no error)"=w1353) -> ("fd out"=w1356:i32, "return value"=w1355:i32, "error out"=w1354:errorcluster)  [unwired: 10 out]
              n434 = Unbundle By Name(w1354) -> ("status"=w1361:bool)
              n435 = case shown="False" w1361 {
                tunnel: w1360 -> [w1372 _]
                frame False {
                  n436 = call "DHE_GetControllerStatus.vi"() -> ("ControllerStatus"=w1371:T5)  [unwired: 11 out]
                  n437 = Bundle By Name(cluster=w1371, "artifdata"=w1372) -> (w1370:T5)
                  n438 = call "DHE_SetControllerParams.vi"("ControllerStatus"=w1370) -> ()  [unwired: 1 in, 10 out]
                }
                frame True {
                }
              }
            }
            frame "artifpattern" {
              n439 = call "DHE_GetArtifPatterns.vi"() -> ("DHE_ArtifPatterns"=w1382:string)  [unwired: 9 out]
              n440 = Scan From String(format string="%s", input string=w1376) -> (remaining string=w1384:string, output 1=w1378:string)  [unwired: 2 in, 3 out]
              n441 = Scan From String(format string="%d", input string=w1376) -> (error out=w1373:errorcluster, output 1=w1374:i32)  [unwired: 2 in, 3 out]
              n442 = call "CMN_Str2Arr.vi"("separator"=",", "string in"=w1382) -> ("Array out"=w1380:string[])  [unwired: 2 in, 7 out]
              n443 = Match First String(2:w1380, 3:w1378) -> (0:w1379:i32)  [unwired: 1 out]
              n444 = Greater Or Equal To 0?(x=w1379) -> (x >= 0?=w1377:bool)
              n445 = case shown="False" w1377 {
                tunnel: w1383 -> [w1393 w1420]
                tunnel: [w1397 w1419] -> w1390
                tunnel: [w1392 w1418] -> w1389
                tunnel: w1388 -> [w1391 w1416]
                tunnel: [w1398 w1417] -> w1387
                tunnel: w1384 -> [w1394 w1412]
                tunnel: w1379 -> [_ w1415]
                tunnel: w1376 -> [_ _]
                tunnel: w1374 -> [w1395 _]
                tunnel: w1373 -> [w1396 _]
                frame False {
                  n446 = case shown="No Error" w1396 {
                    tunnel: [w1401 errorcluster {"status"=TRUE, "code"=-22, "source"="ERROR unknown pattern"} ("error out")] -> w1398
                    tunnel: [w1402 -22 ("return value")] -> w1397
                    tunnel: w1395 -> [w1406 _]
                    tunnel: w1394 -> [w1405 _]
                    tunnel: w1393 -> [w1404 w1408]
                    tunnel: [w1403 w1408] -> w1392
                    tunnel: w1391 -> [w1399 _]
                    frame No Error {
                      (unwired) "%d" ("format string")
                      n447 = Format Into String(w1406) -> (resulting string=w1407:string)  [unwired: 3 in, 1 out]
                      n448 = Concatenate Strings(w1407, w1405) -> (w1400:string)
                      n449 = call "DHE_set_artifpattern.vi"("fd"=w1404, "artifpattern"=w1400, "error in (no error)"=w1399) -> ("fd out"=w1403:i32, "return value"=w1402:i32, "error out"=w1401:errorcluster)  [unwired: 10 out]
                    }
                    frame Error {
                    }
                  }
                }
                frame True {
                  n450 = Format Into String(format string="%d", w1415) -> (resulting string=w1413:string)  [unwired: 2 in, 1 out]
                  n451 = Concatenate Strings(w1413, w1412) -> (w1411:string)
                  n452 = call "DHE_set_artifpattern.vi"("fd"=w1420, "artifpattern"=w1411, "error in (no error)"=w1416) -> ("fd out"=w1418:i32, "return value"=w1419:i32, "error out"=w1417:errorcluster)  [unwired: 10 out]
                }
              }
              n453 = case shown="No Error" w1387 {
                tunnel: w1378 -> [w1421 _]
                tunnel: w1386 -> [w1424 _]
                frame No Error {
                  n454 = call-poly "DatabaseHand_Set.vi"("group"="dhe", "name"="artifpatt", "value"=w1421, "Database RefNum in"=w1424) -> ()  [unwired: 4 in, 4 out]
                }
                frame Error {
                }
              }
            }
            frame "autoshutter" {
              n455 = call "DHE_ParseAutoshutterCmd.vi"("error in (no error)"=w1430, "argument"=w1425, "fd"=w1429) -> ("error out"=w1427:errorcluster, "return value"=w1426:i32, "fd out"=w1428:i32)  [unwired: 6 out]
            }
            frame "autoclear" {
              n456 = Scan From String(format string="%s" ("Format String"), input string=w1438) -> (output 1=w1441:string)  [unwired: 2 in, 4 out]
              n457 = To Lower Case(string=w1441) -> (all lower case string=w1431:string)
              n458 = case shown="\"on\", \"true\", \"yes\"" w1431 {
                tunnel: [0 1] -> w1440
                tunnel: [FALSE TRUE] -> w1433
                frame Default {
                }
                frame "on", "true", "yes" {
                }
              }
              n459 = call "DHE_autoclear.vi"("fd"=w1437, "flag"=w1440, "error in (no error)"=w1439) -> ("fd out"=w1436:i32, "return value"=w1434:i32, "error out"=w1435:errorcluster)  [unwired: 10 out]
              n460 = Unbundle By Name(w1435) -> ("status"=w1432:bool)
              n461 = case shown="False" w1432 {
                tunnel: w1433 -> [w1445 _]
                frame False {
                  n462 = call "DHE_GetControllerStatus.vi"() -> ("ControllerStatus"=w1444:T5)  [unwired: 11 out]
                  n463 = Bundle By Name(cluster=w1444, "autoclear"=w1445) -> (w1443:T5)
                  n464 = call "DHE_SetControllerParams.vi"("ControllerStatus"=w1443) -> ()  [unwired: 1 in, 10 out]
                }
                frame True {
                }
              }
            }
            frame "autohandleclear", "handleclear" {
              n465 = Scan From String(format string="%s" ("Format String"), input string=w1458) -> (output 1=w1459:string)  [unwired: 2 in, 4 out]
              n466 = To Lower Case(string=w1459) -> (all lower case string=w1457:string)
              n467 = case shown="Default" w1457 {
                tunnel: [w1471 TRUE FALSE] -> w1450
                tunnel: [w1471 TRUE TRUE] -> w1451
                frame Default {
                  w1471 = FALSE
                }
                frame "1", "on", "true", "yes" {
                }
                frame "0", "false", "no", "off" {
                }
              }
              n468 = case shown="True" w1451 {
                tunnel: w1450 -> [_ w1470]
                tunnel: w1456 -> [_ w1469]
                tunnel: w1453 -> [w1465 w1466]
                tunnel: [w1464 w1466] -> w1452
                frame False {
                  n469 = Bundle By Name(cluster=w1465, "status"=TRUE, "code"=-22, "source"="ERROR <on | off>") -> (w1464:errorcluster)
                }
                frame True {
                  n470 = call-poly "DatabaseHand_Set.vi"("group"="dhe", "name"="autohandleclear", "value"=w1470, "Database RefNum in"=w1469) -> ()  [unwired: 4 in, 4 out]
                }
              }
            }
            frame "arm" {
              n471 = Scan From String(format string="%s" ("Format String"), input string=w1484) -> (output 1=w1487:string)  [unwired: 2 in, 4 out]
              n472 = To Lower Case(string=w1487) -> (all lower case string=w1477:string)
              n473 = case shown="\"1\", \"enable\", \"on\", \"true\", \"yes\"" w1477 {
                tunnel: [0 1] -> w1486
                tunnel: [FALSE TRUE] -> w1479
                frame Default {
                }
                frame "1", "enable", "on", "true", "yes" {
                }
              }
              n474 = call "DHE_arm.vi"("fd"=w1483, "flag"=w1486, "error in (no error)"=w1485) -> ("fd out"=w1482:i32, "return value"=w1480:i32, "error out"=w1481:errorcluster)  [unwired: 10 out]
              n475 = Unbundle By Name(w1481) -> ("status"=w1478:bool)
              n476 = case shown="False" w1478 {
                tunnel: w1479 -> [w1489 _]
                tunnel: w1476 -> [w1492 _]
                frame False {
                  n477 = call-poly "DatabaseHand_Set.vi"("group"="dhe", "name"="armed", "value"=w1489, "Database RefNum in"=w1492) -> ()  [unwired: 4 in, 4 out]
                }
                frame True {
                }
              }
            }
            frame "sampling" {
              n478 = call "DHE_SetSampling.vi"("DBS Ref"=w1498, "error in"=w1503, "sampling type"=w1497, "fd"=w1499) -> ("error out"=w1502:errorcluster, "read value"=w1501:i32, "fd"=w1500:i32)  [unwired: 5 out]
            }
            frame "size" {
              n479 = Scan From String(format string="%d %d" ("Format String"), input string=w1504) -> (output 1=w1511:i32, output 2=w1510:i32)  [unwired: 2 in, 5 out]
              n480 = call "DHE_dimensions.vi"("fd"=w1508, "Columns"=w1511, "Rows"=w1510, "error in (no error)"=w1509) -> ("fd out"=w1507:i32, "return value"=w1506:i32, "error out"=w1505:errorcluster)  [unwired: 9 out]
              n481 = call "DHE_SetSizeVals.vi"("error in"=w1505, "ytotsize"=w1510, "xtotsize"=w1511) -> ()  [unwired: 9 out]
            }
            frame "power" {
              n482 = Scan From String(format string="%s" ("Format String"), input string=w1522) -> (output 1=w1523:string)  [unwired: 2 in, 4 out]
              n483 = To Lower Case(string=w1523) -> (all lower case string=w1513:string)
              n484 = case shown="Default" w1513 {
                tunnel: [0 1] -> w1514
                frame Default {
                }
                frame "on", "true", "yes" {
                }
              }
              n485 = call "DHE_power.vi"("fd"=w1521, "flag"=w1514, "error in (no error)"=w1520) -> ("fd out"=w1516:i32, "return value"=w1515:i32, "error out"=w1519:errorcluster)  [unwired: 10 out]
              n486 = Unbundle By Name(w1519) -> ("status"=w1518:bool)
              n487 = case shown="False" w1518 {
                tunnel: w1517 -> [w1530 _]
                tunnel: w1514 -> [w1528 _]
                frame False {
                  n488 = Greater Than 0?(x=w1528) -> (x > 0?=w1527:bool)
                  n489 = Bundle By Name(cluster=w1530, "power"=w1527) -> (w1529:T5)
                  n490 = call "DHE_SetControllerParams.vi"("ControllerStatus"=w1529) -> ()  [unwired: 1 in, 10 out]
                }
                frame True {
                }
              }
            }
            frame "gain" {
              n491 = call "DHE_set_gain.vi"("fd"=w1539, "gain"=w1531, "error in (no error)"=w1538) -> ("fd out"=w1534:i32, "return value"=w1533:i32, "error out"=w1537:errorcluster)  [unwired: 10 out]
              n492 = Unbundle By Name(w1537) -> ("status"=w1536:bool)
              n493 = case shown="False" w1536 {
                tunnel: w1535 -> [w1544 _]
                tunnel: w1531 -> [w1541 _]
                frame False {
                  n494 = Scan From String(format string="%d", input string=w1541) -> (output 1=w1540:i32)  [unwired: 2 in, 4 out]
                  n495 = Bundle By Name(cluster=w1544, "gain"=w1540) -> (w1543:T5)
                  n496 = call "DHE_SetControllerParams.vi"("ControllerStatus"=w1543) -> ()  [unwired: 1 in, 10 out]
                }
                frame True {
                }
              }
              n497 = call <vilib>:"Trim Whitespace.vi"("string"=w1531) -> ("trimmed string"=w1532:string)  [unwired: 1 in]
            }
            frame "pixtime", "speed" {
              n498 = Scan From String(format string="%g" ("Format String"), input string=w1550) -> (output 1=w1551:dbl)  [unwired: 2 in, 4 out]
              n499 = Equal?(x=w1547, y="speed") -> (x = y?=w1545:bool)
              n500 = case shown="False" w1545 {
                tunnel: w1558 -> [w1566 w1573]
                tunnel: w1557 -> [w1565 w1572]
                tunnel: [w1564 w1571] -> w1556
                tunnel: [w1563 w1570] -> w1555
                tunnel: [w1562 w1569] -> w1553
                tunnel: [w1561 w1568] -> w1552
                tunnel: w1551 -> [w1560 w1567]
                frame True {
                  n501 = call "DHE_set_speed.vi"("fd"=w1566, "speed"=w1560, "error in (no error)"=w1565) -> ("fd out"=w1562:i32, "return value"=w1561:i32, "error out"=w1564:errorcluster)  [unwired: 10 out]
                  n502 = Unbundle By Name(w1564) -> ("status"=w1563:bool)
                }
                frame False {
                  n503 = call "DHE_set_pixtime.vi"("fd"=w1573, "time"=w1567, "error in (no error)"=w1572) -> ("fd out"=w1569:i32, "return value"=w1568:i32, "error out"=w1571:errorcluster)  [unwired: 10 out]
                  n504 = Unbundle By Name(w1571) -> ("status"=w1570:bool)
                }
              }
              n505 = case shown="False" w1555 {
                tunnel: w1554 -> [w1593 _]
                tunnel: w1551 -> [w1592 _]
                tunnel: w1548 -> [w1574 _]
                tunnel: w1545 -> [w1575 _]
                frame False {
                  # "recalc readtime"
                  n506 = call "DHE_GetReadMode.vi"() -> ("DHE_ReadMode"=w1589:string)  [unwired: 9 out]
                  n507 = call "DHE_GetDetXYSize.vi"() -> ("DHE_DetYsize"=w1590:i32, "DHE_DetXsize"=w1591:i32)  [unwired: 8 out]
                  n508 = call "GEOM_GetFPA.vi"("readmode"=w1589) -> ("CorrectedFPACoord"=w1588:T9, "amplifiers"=w1581:T10[], "numyamps"=w1584:i32, "numxamps"=w1583:i32)  [unwired: 2 in, 5 out]
                  n509 = case shown="False" w1575 {
                    tunnel: w1593 -> [_ w1600]
                    tunnel: w1592 -> [w1594 w1599]
                    tunnel: w1574 -> [w1597 _]
                    frame False {
                      n510 = call-poly "DatabaseHand_Set.vi"("group"="dhe", "name"="pixtime", "value"=w1594, "Database RefNum in"=w1597) -> ()  [unwired: 4 in, 4 out]
                    }
                    frame True {
                      n511 = Bundle By Name(cluster=w1600, "speed"=w1599) -> (w1598:T5)
                      n512 = call "DHE_SetControllerParams.vi"("ControllerStatus"=w1598) -> ()  [unwired: 1 in, 10 out]
                    }
                  }
                  n513 = Unbundle By Name(w1588) -> ("totxsize"=w1587:i32, "totysize"=w1586:i32)
                  n514 = Index Array(array=w1581, index=0) -> (element=w1580:T10)
                  n515 = Array Size(array=w1581) -> (size(s)=w1585:i32)
                  n516 = Unbundle By Name(w1580) -> ("Corr ROI"=w1579:T12)
                  n517 = Index Array(array=w1579, index=0) -> (element=w1577:T13)
                  n518 = Unbundle By Name(w1577) -> ("ystart"=w1576:u32)
                  n519 = call "DHE_SetTiming.vi"("num of Y amps"=w1584, "num of X amps"=w1583, "yroi start"=w1576, "roi rows"=w1586, "Num of amps"=w1585, "roi cols"=w1587, "totysize"=w1590, "totxsize"=w1591, "Database RefNum out"=w1574) -> ()  [unwired: 1 in, 2 out]
                }
                frame True {
                }
              }
              n520 = call <vilib>:"Trim Whitespace.vi"("string"=w1550) -> ("trimmed string"=w1549:string)  [unwired: 1 in]
            }
            frame "deftiming", "timing" {
              n521 = Scan From String(format string="%s %g" ("Format String"), input string=w1613) -> (output 1=w1605:string, output 2=w1606:dbl)  [unwired: 2 in, 5 out]
              n522 = To Lower Case(string=w1605) -> (all lower case string=w1601:string)
              n523 = call "DHE_GetTimingInfo.vi"("Database RefNum out"=w1608) -> ("Timing"=w1609:T8)  [unwired: 10 out]
              n524 = Greater Or Equal To 0?(x=w1606) -> (x >= 0?=w1611:bool)
              n525 = case shown="True" w1611 {
                selector: w1611 -> [w1616 w1618]
                tunnel: [w1616 w1617] -> w1610
                tunnel: w1609 -> [_ w1622]
                tunnel: w1606 -> [_ w1621]
                tunnel: w1608 -> [_ w1620]
                tunnel: w1601 -> [_ w1619]
                frame False {
                }
                frame True {
                  n526 = case shown="\"known_overhead\", \"overhead\"" w1619 {
                    tunnel: w1622 -> [_ w1628 w1633 w1638 w1643 w1648 w1653]
                    tunnel: w1621 -> [_ w1627 w1632 w1637 w1642 w1647 w1652]
                    tunnel: w1620 -> [_ w1626 w1631 w1636 w1641 w1646 w1651]
                    tunnel: w1618 -> [_ w1624 w1629 w1634 w1639 w1644 w1649]
                    tunnel: [FALSE w1624 w1629 w1634 w1639 w1644 w1649] -> w1617
                    frame Default {
                    }
                    frame "pixeltime", "pixtime" {
                      n527 = Bundle By Name(cluster=w1628, "PixelTime"=w1627) -> (w1625:T8)
                      n528 = call "DHE_SetTimingInfo.vi"("Timing"=w1625, "Database RefNum out"=w1626) -> ()  [unwired: 10 out]
                    }
                    frame "skippixel" {
                      n529 = Bundle By Name(cluster=w1633, "SkipPixel"=w1632) -> (w1630:T8)
                      n530 = call "DHE_SetTimingInfo.vi"("Timing"=w1630, "Database RefNum out"=w1631) -> ()  [unwired: 10 out]
                    }
                    frame "skiprow" {
                      n531 = Bundle By Name(cluster=w1638, "SkipRow"=w1637) -> (w1635:T8)
                      n532 = call "DHE_SetTimingInfo.vi"("Timing"=w1635, "Database RefNum out"=w1636) -> ()  [unwired: 10 out]
                    }
                    frame "shiftrow" {
                      n533 = Bundle By Name(cluster=w1643, "ShiftRow"=w1642) -> (w1640:T8)
                      n534 = call "DHE_SetTimingInfo.vi"("Timing"=w1640, "Database RefNum out"=w1641) -> ()  [unwired: 10 out]
                    }
                    frame "shiftedpix" {
                      n535 = Bundle By Name(cluster=w1648, "ShiftedPix"=w1647) -> (w1645:T8)
                      n536 = call "DHE_SetTimingInfo.vi"("Timing"=w1645, "Database RefNum out"=w1646) -> ()  [unwired: 10 out]
                    }
                    frame "known_overhead", "overhead" {
                      n537 = Bundle By Name(cluster=w1653, "known_overhead"=w1652) -> (w1650:T8)
                      n538 = call "DHE_SetTimingInfo.vi"("Timing"=w1650, "Database RefNum out"=w1651) -> ()  [unwired: 10 out]
                    }
                  }
                }
              }
              n539 = case shown="True" w1610 {
                tunnel: w1614 -> [_ _]
                tunnel: w1606 -> [_ w1680]
                tunnel: w1608 -> [_ w1663]
                tunnel: w1604 -> [w1658 w1660]
                tunnel: [w1657 w1660] -> w1603
                tunnel: [w1654 0 ("code")] -> w1602
                frame False {
                  w1654 = -22 ("code")
                  n540 = Bundle By Name(cluster=w1658, "status"=TRUE, "code"=w1654, "source"="ERROR unknow timing param or bad value") -> (w1657:errorcluster)
                }
                frame True {
                  # "recalc readtime"
                  n541 = call "DHE_GetReadMode.vi"() -> ("DHE_ReadMode"=w1677:string)  [unwired: 9 out]
                  n542 = call "DHE_GetDetXYSize.vi"() -> ("DHE_DetYsize"=w1678:i32, "DHE_DetXsize"=w1679:i32)  [unwired: 8 out]
                  n543 = call "GEOM_GetFPA.vi"("readmode"=w1677) -> ("CorrectedFPACoord"=w1676:T9, "amplifiers"=w1669:T10[], "numyamps"=w1672:i32, "numxamps"=w1671:i32)  [unwired: 2 in, 5 out]
                  n544 = Unbundle By Name(w1676) -> ("totxsize"=w1675:i32, "totysize"=w1674:i32)
                  n545 = Index Array(array=w1669, index=0) -> (element=w1668:T10)
                  n546 = Array Size(array=w1669) -> (size(s)=w1673:i32)
                  n547 = Unbundle By Name(w1668) -> ("Corr ROI"=w1667:T12)
                  n548 = call-poly "DatabaseHand_Set.vi"("group"="dhe", "name"="defpixtime", "value"=w1680, "Database RefNum in"=w1663) -> ()  [unwired: 4 in, 4 out]
                  n549 = Index Array(array=w1667, index=0) -> (element=w1665:T13)
                  n550 = Unbundle By Name(w1665) -> ("ystart"=w1664:u32)
                  n551 = call "DHE_SetTiming.vi"("num of Y amps"=w1672, "num of X amps"=w1671, "yroi start"=w1664, "roi rows"=w1674, "Num of amps"=w1673, "roi cols"=w1675, "totysize"=w1678, "totxsize"=w1679, "Database RefNum out"=w1663) -> ()  [unwired: 1 in, 2 out]
                }
              }
              n552 = call <vilib>:"Trim Whitespace.vi"("string"=w1613) -> ("trimmed string"=w1612:string)  [unwired: 1 in]
            }
            frame "expcode", "expvector" {
              n553 = Scan From String(format string="%d" ("Format String"), input string=w1683) -> (output 1=w1684:i32)  [unwired: 2 in, 4 out]
              n554 = call "DHE_set_expCode.vi"("fd"=w1691, "code"=w1684, "error in (no error)"=w1690) -> ("fd out"=w1686:i32, "return value"=w1685:i32, "error out"=w1689:errorcluster)  [unwired: 10 out]
              n555 = Unbundle By Name(w1689) -> ("status"=w1688:bool)
              n556 = case shown="False" w1688 {
                tunnel: w1687 -> [_ _]
                tunnel: w1684 -> [w1693 _]
                tunnel: w1681 -> [w1696 _]
                frame False {
                  n557 = call-poly "DatabaseHand_Set.vi"("group"="dhe", "name"="expcode", "value"=w1693, "Database RefNum in"=w1696) -> ()  [unwired: 4 in, 4 out]
                }
                frame True {
                }
              }
              n558 = call <vilib>:"Trim Whitespace.vi"("string"=w1683) -> ("trimmed string"=w1682:string)  [unwired: 1 in]
            }
            frame "expasync" {
              n559 = Scan From String(format string="%s", input string=w1698) -> (output 1=w1703:string)  [unwired: 2 in, 4 out]
              n560 = call <vilib>:"Trim Whitespace.vi"("string"=w1698) -> ("trimmed string"=w1697:string)  [unwired: 1 in]
              n561 = To Lower Case(string=w1703) -> (all lower case string=w1702:string)
              n562 = case shown="\"false\", \"no\", \"off\"" w1702 {
                tunnel: w1701 -> [w1710 w1713 w1716]
                tunnel: [w1709 w1713 w1716] -> w1700
                tunnel: [w1707 0 ("code") 0 ("code")] -> w1699
                frame Default {
                  w1707 = -22 ("code")
                  n563 = Bundle By Name(cluster=w1710, "status"=TRUE, "code"=w1707, "source"="ERROR <on | off>") -> (w1709:errorcluster)
                }
                frame "on", "true", "yes" {
                  n564 = call "DHE_SetAsyncExp.vi"("DHE_asyncexp"=TRUE) -> ()  [unwired: 9 out]
                }
                frame "false", "no", "off" {
                  n565 = call "DHE_SetAsyncExp.vi"("DHE_asyncexp"=FALSE) -> ()  [unwired: 9 out]
                }
              }
            }
            frame "appendid" {
              n566 = Scan From String(format string="%s", input string=w1718) -> (output 1=w1723:string)  [unwired: 2 in, 4 out]
              n567 = call <vilib>:"Trim Whitespace.vi"("string"=w1718) -> ("trimmed string"=w1717:string)  [unwired: 1 in]
              n568 = To Lower Case(string=w1723) -> (all lower case string=w1722:string)
              n569 = case shown="\"on\", \"true\", \"yes\"" w1722 {
                tunnel: w1721 -> [w1730 w1733 w1736]
                tunnel: [w1729 w1733 w1736] -> w1720
                tunnel: [w1727 0 ("code") 0 ("code")] -> w1719
                frame Default {
                  w1727 = -22 ("code")
                  n570 = Bundle By Name(cluster=w1730, "status"=TRUE, "code"=w1727, "source"="ERROR <on | off>") -> (w1729:errorcluster)
                }
                frame "on", "true", "yes" {
                  n571 = call "DHE_SetAppendID.vi"("DHE_appendid"=TRUE ("DHE_asyncexp")) -> ()  [unwired: 9 out]
                }
                frame "false", "no", "off" {
                  n572 = call "DHE_SetAppendID.vi"("DHE_appendid"=FALSE ("DHE_asyncexp")) -> ()  [unwired: 9 out]
                }
              }
            }
            frame "shutter" {
              n573 = Scan From String(format string="%s" ("Format String"), input string=w1738) -> (remaining string=w1740:string, output 1=w1751:string)  [unwired: 2 in, 3 out]
              n574 = To Lower Case(string=w1751) -> (all lower case string=w1749:string)
              n575 = case shown="\"1\", \"on\", \"open\", \"true\", \"yes\"" w1749 {
                tunnel: [0 w1787 0 0] -> w1742
                tunnel: [0 w1787 1 2] -> w1741
                frame Default {
                }
                frame "1", "on", "open", "true", "yes" {
                  w1787 = 1
                }
                frame "0", "close", "false", "no", "off" {
                }
                frame "type" {
                }
              }
              n576 = case shown="2" w1741 {
                tunnel: w1748 -> [w1757 w1764 w1779]
                tunnel: [w1757 w1763 w1778] -> w1747
                tunnel: w1746 -> [w1756 w1762 w1777]
                tunnel: [w1752 w1761 w1776] -> w1745
                tunnel: [w1754 w1760 w1775] -> w1744
                tunnel: w1743 -> [_ w1759 w1774]
                tunnel: w1742 -> [_ w1758 _]
                tunnel: w1740 -> [_ _ w1773]
                tunnel: w1739 -> [_ _ w1771]
                frame 0, Default {
                  w1754 = -22 ("return value")
                  n577 = Bundle By Name(cluster=w1756, "status"=TRUE, "code"=w1754, "source"="ERROR <open | close | type <type>") -> (w1752:errorcluster)
                }
                frame 1 {
                  n578 = call "DHE_move_shutter.vi"("fd"=w1764, "flag"=w1758, "error in (no error)"=w1762) -> ("fd out"=w1763:i32, "return value"=w1760:i32, "error out"=w1761:errorcluster)  [unwired: 10 out]
                  n579 = Unbundle By Name(w1761) -> ("status"=w1765:bool)
                  n580 = case shown="False" w1765 {
                    tunnel: w1759 -> [w1768 _]
                    tunnel: w1758 -> [w1767 _]
                    frame False {
                      n581 = Greater Than 0?(x=w1767) -> (x > 0?=w1766:bool)
                      n582 = Bundle By Name(cluster=w1768, "shutter"=w1766) -> (w1769:T5)
                      n583 = call "DHE_SetControllerParams.vi"("ControllerStatus"=w1769) -> ()  [unwired: 1 in, 10 out]
                    }
                    frame True {
                    }
                  }
                }
                frame 2 {
                  n584 = Scan From String(format string="%s", input string=w1773) -> (output 1=w1770:string)  [unwired: 2 in, 4 out]
                  n585 = call "DHE_set_shutter_type.vi"("fd"=w1779, "type"=w1770, "error in (no error)"=w1777) -> ("fd out"=w1778:i32, "return value"=w1775:i32, "error out"=w1776:errorcluster)  [unwired: 10 out]
                  n586 = Unbundle By Name(w1776) -> ("status"=w1780:bool)
                  n587 = case shown="False" w1780 {
                    tunnel: w1774 -> [_ _]
                    tunnel: w1771 -> [w1783 _]
                    tunnel: w1770 -> [w1782 _]
                    frame False {
                      n588 = call-poly "DatabaseHand_Set.vi"("group"="dhe", "name"="shutt_type", "value"=w1782, "Database RefNum in"=w1783) -> ()  [unwired: 4 in, 4 out]
                    }
                    frame True {
                    }
                  }
                }
              }
              n589 = call <vilib>:"Trim Whitespace.vi"("string"=w1738) -> ("trimmed string"=w1737:string)  [unwired: 1 in]
            }
            frame "config", "state" {
              w1794 = -1 ("code")
              n590 = Bundle By Name(cluster=w1796, "status"=TRUE, "code"=w1794, "source"="ERR: read-only parameter") -> (w1795:errorcluster)
            }
          }
        }
        frame "outputtype" {
          n591 = Scan From String(format string="%s" ("Format String"), input string=w1808) -> (output 1=w1802:string)  [unwired: 2 in, 4 out]
          n592 = call "CMN_TrimStringWhitespace.vi"("Both Ends?(T)"=TRUE ("Both Ends?(F)"), "string"=w1802) -> ("trimmed string"=w1799:string)  [unwired: 8 out]
          n593 = case shown="\"16_bits\"" w1799 {
            selector: w1799 -> [w1811 w1817]
            tunnel: w1806 -> [w1816 w1821]
            tunnel: [w1815 w1821] -> w1805
            tunnel: [w1813 0 ("code")] -> w1804
            tunnel: w1800 -> [_ w1819]
            frame Default {
              w1813 = -22 ("code")
              n594 = Concatenate Strings("SDSU-IISettings: Unknown " ("source"), w1811, "OutputType ") -> (w1809:string)
              n595 = Bundle By Name(cluster=w1816, "status"=TRUE, "code"=w1813, "source"=w1809) -> (w1815:errorcluster)
            }
            frame "16_bits" {
              n596 = Bundle By Name(cluster=w1819, "datatype"=w1817) -> (w1818:T5)
              n597 = call "DHE_SetControllerParams.vi"("ControllerStatus"=w1818) -> ()  [unwired: 1 in, 10 out]
            }
          }
        }
        frame "delay" {
          n598 = Scan From String(format string="%d", input string=w1827) -> (output 1=w1825:i32)  [unwired: 2 in, 4 out]
          n599 = In Range and Coerce(upper limit=20000, x=w1825, lower limit=1) -> (coerced(x)=w1822:i32)  [unwired: 1 out]
          n600 = Wait (ms)(milliseconds to wait=w1822) -> ()  [unwired: 1 out]
        }
        frame "macro_dir", "macrodir" {
          n601 = Scan From String(format string="%s" ("Format String"), input string=w1836) -> (output 1=w1838:string)  [unwired: 2 in, 4 out]
          n602 = call "CMN_TrimStringWhitespace.vi"("Both Ends?(T)"=TRUE ("Both Ends?(F)"), "string"=w1838) -> ("trimmed string"=w1832:string)  [unwired: 8 out]
          n603 = String To Path(string=w1832) -> (path=w1837:path)
          n604 = call "DHE_SetMacroDir.vi"("DHE_MacroDir"=w1837) -> ()  [unwired: 9 out]
        }
        frame "init_macro", "initmacro" {
          n605 = Scan From String(format string="%s" ("Format String"), input string=w1846) -> (output 1=w1847:string)  [unwired: 2 in, 4 out]
          n606 = call "CMN_TrimStringWhitespace.vi"("Both Ends?(T)"=TRUE ("Both Ends?(F)"), "string"=w1847) -> ("trimmed string"=w1842:string)  [unwired: 8 out]
          n607 = String To Path(string=w1842) -> (path=w1841:path)
          n608 = call "DHE_SetInitMacro.vi"("DHE_InitMacro"=w1841) -> ()  [unwired: 9 out]
        }
        frame "normalize", "normalize_coadd", "normalize_coadds" {
          n609 = Scan From String(format string="%s" ("Format String"), input string=w1850) -> (output 1=w1861:string)  [unwired: 2 in, 4 out]
          n610 = call "CMN_TrimStringWhitespace.vi"("Both Ends?(T)"=TRUE ("Both Ends?(F)"), "string"=w1861) -> ("trimmed string"=w1859:string)  [unwired: 8 out]
          n611 = To Lower Case(string=w1859) -> (all lower case string=w1858:string)
          n612 = case shown="\"on\", \"true\", \"yes\"" w1858 {
            tunnel: w1854 -> [w1868 w1874 w1879]
            tunnel: [w1868 w1874 w1878] -> w1853
            tunnel: [0 0 w1875] -> w1852
            tunnel: w1855 -> [w1866 w1871 _]
            tunnel: "improc" ("group") -> [w1864 w1870 _]
            tunnel: "normalize_coadds" ("value") -> [w1863 w1869 _]
            frame "on", "true", "yes" {
              n613 = call-poly "DatabaseHand_Set.vi"("group"=w1864, "name"=w1863, "value"=TRUE ("Normalize"), "Database RefNum in"=w1866) -> ()  [unwired: 4 in, 4 out]
            }
            frame "false", "no", "off" {
              n614 = call-poly "DatabaseHand_Set.vi"("group"=w1870, "name"=w1869, "value"=FALSE ("Normalize"), "Database RefNum in"=w1871) -> ()  [unwired: 4 in, 4 out]
            }
            frame Default {
              w1875 = -22 ("code")
              n615 = Bundle By Name(cluster=w1879, "status"=TRUE, "code"=w1875, "source"="ERROR: Normalize <on | off>") -> (w1878:errorcluster)
            }
          }
        }
        frame "detector_format", "detformat" {
          n616 = Scan From String(format string="%s" ("Format String"), input string=w1883) -> (output 1=w1888:string)  [unwired: 2 in, 4 out]
          n617 = Match Pattern(string=w1888, regular expression="[x,X]") -> (offset past match=w1881:i32)  [unwired: 4 out]
          n618 = Greater Or Equal To 0?(x=w1881) -> (x >= 0?=w1880:bool)
          n619 = To Lower Case(string=w1888) -> (all lower case string=w1895:string)
          n620 = Search 1D Array(1D array=w1884, element="-default") -> (index of element=w1898:i32)  [unwired: 1 out]
          n621 = Equal?(x=w1895, y="default") -> (x = y?=w1894:bool)
          n622 = Greater Or Equal To 0?(x=w1898) -> (x >= 0?=w1897:bool)
          n623 = Or(x=w1894, y=w1897) -> (x .or. y?=w1893:bool)
          n624 = case shown="False" w1893 {
            tunnel: w1889 -> [w1905 w1929]
            tunnel: [w1909 w1930] -> w1885
            tunnel: w1891 -> [w1906 w1928]
            tunnel: [w1908 w1926] -> w1887
            tunnel: [w1907 w1925] -> w1886
            tunnel: w1890 -> [w1904 w1927]
            tunnel: w1888 -> [w1903 _]
            tunnel: FALSE ("forece init") -> [w1902 w1924]
            tunnel: w1880 -> [w1901 _]
            frame False {
              n625 = case shown="True" w1901 {
                tunnel: [w1912 w1923] -> w1909
                tunnel: [w1911 w1922] -> w1908
                tunnel: [w1910 w1921] -> w1907
                tunnel: w1906 -> [w1911 w1920]
                tunnel: w1905 -> [w1913 w1919]
                tunnel: w1904 -> [_ w1916]
                tunnel: w1903 -> [_ w1918]
                tunnel: w1902 -> [_ w1917]
                frame False {
                  w1910 = -22 ("code")
                  n626 = Bundle By Name(cluster=w1913, "status"=TRUE, "code"=w1910, "source"="ERROR wrong format (try colsxrows)") -> (w1912:errorcluster)
                }
                frame True {
                  # "start geiometry with the \"override value\" provided`"
                  n627 = call "DHE_InitGeometry.vi"("refnum"=w1920, "override format"=w1918, "error in (no error)"=w1919, "Database RefNum out"=w1916, "forece init"=w1917) -> ("fd out"=w1922:i32, "return value"=w1921:i32, "error out"=w1923:errorcluster)  [unwired: 8 out]
                }
              }
            }
            frame True {
              # "init geometry with default values\n(stated on the DET_DATABASE module)"
              n628 = call "DHE_InitGeometry.vi"("refnum"=w1928, "override format"="", "error in (no error)"=w1929, "Database RefNum out"=w1927, "forece init"=w1924) -> ("fd out"=w1926:i32, "return value"=w1925:i32, "error out"=w1930:errorcluster)  [unwired: 8 out]
            }
          }
        }
        frame "memrule" {
          n629 = call <vilib>:"Trim Whitespace.vi"("string"=w1935) -> ("trimmed string"=w1934:string)  [unwired: 1 in]
          n630 = To Lower Case(string=w1934) -> (all lower case string=w1933:string)
          n631 = call-poly "DatabaseHand_Set.vi"("group"="dhe", "name"="memrule", "value"=w1933, "Database RefNum in"=w1932) -> ()  [unwired: 4 in, 4 out]
        }
        frame "interlock", "interlocks" {
          n632 = Scan From String(format string="%s", input string=w1948) -> (remaining string=w1945:string, output 1=w1946:string)  [unwired: 2 in, 3 out]
          n633 = call <vilib>:"Trim Whitespace.vi"("string"=w1945) -> ("trimmed string"=w1944:string)  [unwired: 1 in]
          n634 = case shown="\"add\", \"edit\"" w1946 {
            tunnel: w1944 -> [_ w1960 w1964 w1969]
            tunnel: [w1953 w1959 w1963 w1968] -> w1943
            tunnel: w1942 -> [w1952 w1958 w1962 w1967]
            tunnel: [w1951 w1957 w1961 w1966] -> w1941
            frame Default {
              w1953 = "ERROR interlock <add | delete> <state> <command>" ("response")
              n635 = Bundle By Name(cluster=w1952, "status"=TRUE, "code"=-22, "source"=w1953) -> (w1951:errorcluster)
            }
            frame "add", "edit" {
              n636 = call "DHE_InterlockMngr.vi"("error in (no error)"=w1958, "Enum"=T3."add", "command"=w1960) -> ("error out"=w1957:errorcluster, "response"=w1959:string)  [unwired: 1 in, 6 out]
            }
            frame "delete" {
              n637 = call "DHE_InterlockMngr.vi"("error in (no error)"=w1962, "Enum"=T4."delete", "command"=w1964) -> ("error out"=w1961:errorcluster, "response"=w1963:string)  [unwired: 1 in, 6 out]
            }
            frame "clear", "clearall", "deleteall" {
              n638 = call "DHE_InterlockMngr.vi"("error in (no error)"=w1967, "Enum"=T4."clear all", "command"=w1969) -> ("error out"=w1966:errorcluster, "response"=w1968:string)  [unwired: 1 in, 6 out]
            }
          }
        }
        frame "dbs" {
          n639 = Scan From String(format string="%s %s", input string=w1971) -> (output 1=w1979:string, output 2=w1978:string)  [unwired: 4 in, 3 out]
          n640 = call-poly "DatabaseHand_Get.vi"("name"=w1979, "Database RefNum in"=w1972) -> ("error out"=w1980:errorcluster, "type"=w1977:string)  [unwired: 3 in, 5 out]
          n641 = case shown="No Error" w1980 {
            tunnel: w1972 -> [w1987 _]
            tunnel: w1979 -> [w1986 _]
            tunnel: w1978 -> [w1985 _]
            tunnel: w1977 -> [w1984 _]
            tunnel: [w1983 "ERROR unknow var" ("response")] -> w1976
            frame No Error {
              n642 = call "DHE_DBS_SetByType.vi"("queue?"=FALSE, "type"=w1984, "value"=w1985, "name"=w1986, "Database RefNum"=w1987) -> ("response"=w1983:string)  [unwired: 6 in]
            }
            frame Error {
            }
          }
        }
        frame Default {
          n643 = case shown="\"\", \"?\", \"help\"" w1992 {
            selector: w1992 -> [w2005 _]
            tunnel: w1994 -> [_ _]
            tunnel: [w2005 w2011] -> w1993
            tunnel: [TRUE FALSE] -> w1991
            frame "", "?", "help" {
            }
            frame Default {
              n644 = Scan From String(format string="%s", input string="raw args") -> (remaining string=w2007:string, output 1=w2008:string)  [unwired: 2 in, 3 out]
              n645 = Concatenate Strings("set_" ("string"), w2008, w2007) -> (w2011:string)
            }
          }
          n646 = call "DHE_send_custom.vi"("valid params"=string[] ["image.<..> [?]", "dhe.<..> [?]", "obs.<..> [?]", "macrodir <dir>", "detformat [<colsXrows>] [-default]", "normalize <on | off>"], "error in (no error)"=w1999, "args"=w1993, "fd"=w1996) -> ("error IO"=w1990:errorcluster, "fd out"=w1995:i32)  [unwired: 6 out]
          n647 = Unbundle By Name(w1990) -> ("code"=w1998:i32)
          n648 = case shown="True" w1991 {
            tunnel: w1990 -> [w2000 w2003]
            tunnel: [w2000 w2002] -> w1989
            frame False {
            }
            frame True {
              n649 = Bundle By Name(cluster=w2003, "status"=TRUE) -> (w2002:errorcluster)
            }
          }
        }
      }
      n650 = call "DHE_asyncvarsMgr.vi"("action"=T2."send", "error in (no error)"=w14, "value"=w12, "var"=w13) -> ()  [unwired: 8 out]
    }
    frame Error {
      n651 = Unbundle By Name(w2013) -> ("code"=w2014:i32)
    }
  }
  "Read Value" <- w11
  "refnum out" <- w10
  "error out" <- w4
  n652 = Unbundle By Name(w4) -> ("source"=w2:string)
  n653 = Select(t=w2, s=w4, f="DONE") -> (s? t:f=→"message":string)
